vi "Lab Panel V2.3.vi"() -> ()   [LabVIEW 2013]
uses:
  <vilib>/Platform/TimedLoop/XDataNode/timing_clust.ctl
  <vilib>/Platform/TimedLoop/XDataNode/nitl_modes.ctl
  <vilib>/Platform/TimedLoop/XDataNode/wakeup.ctl
  <vilib>/platform/TimedLoop/XDataNode/XDataNode.xnode
  <vilib>/Platform/TimedLoop/XDataNode/XDNodeRunTimeDep.lvlib
panel:
  out "TEMP update":bool
  out "AI update":bool
  in  "stop":bool
  in  "Tab Control 2":T1(tab)
  out "LAB05-2 (SIG)":T2 {"PF" format="%.2f"; "AMPS" format="%.1f"}
  out "LAB05-1 (SIG)":T2 {"PF" format="%.2f"; "AMPS" format="%.1f"}
  out "LAB04-2 (SIG)":T2 {"PF" format="%.2f"; "AMPS" format="%.1f"}
  out "LAB04-1 (SIG)":T2 {"PF" format="%.2f"; "AMPS" format="%.1f"}
  out "LAB03-2 (SIG)":T2 {"PF" format="%.2f"; "AMPS" format="%.1f"}
  out "LAB03-1 (SIG)":T2 {"PF" format="%.2f"; "AMPS" format="%.1f"}
  out "LAB02-2 (SIG)":T2 {"PF" format="%.2f"; "AMPS" format="%.1f"}
  in  "LAB01-1RUN":bool
  in  "LAB05-1 (O/I)":bool
  in  "LAB05-2 (O/I)":bool
  in  "LAB04-1 (O/I)":bool
  in  "LAB04-2 (O/I)":bool
  in  "LAB02-1 (O/I)":bool
  in  "LAB02-2 (O/I)":bool
  in  "LAB01-2 (O/I)":bool
  in  "LAB01-1 (O/I)":bool
  in  "LAB03-1 (O/I)":bool
  in  "LAB05-2 RUN":bool
  in  "LAB05-1 RUN":bool
  in  "LAB04-2 RUN":bool
  in  "LAB04-1 RUN":bool
  in  "LAB03-2 RUN":bool
  in  "LAB03-1 RUN":bool
  in  "LAB02-2 RUN":bool
  in  "LAB02-1 RUN":bool
  in  "LAB01-2 RUN":bool
  in  "LAB05-2 SELECT":T3(radio)
  in  "LAB05-1 SELECT":T3(radio)
  in  "LAB04-2 SELECT":T3(radio)
  in  "LAB04-1 SELECT":T3(radio)
  in  "LAB03-2 SELECT":T3(radio)
  in  "LAB03-1 SELECT":T3(radio)
  in  "LAB02-2 SELECT":T3(radio)
  in  "LAB02-1 SELECT":T3(radio)
  in  "LAB01-2 SELECT":T3(radio)
  in  "LAB01-1 SELECT":T3(radio)
  in  "LAB03-2 (O/I)":bool
  out "LAB01-1 (SIG)":T2 {"PF" format="%.2f"; "AMPS" format="%.1f"}
  out "LAB01-2 (SIG)":T2 {"PF" format="%.2f"; "AMPS" format="%.1f"}
  out "LAB02-1 (SIG)":T2 {"PF" format="%.2f"; "AMPS" format="%.1f"}
  in  "LAB05 (SETTINGS 1)":T4={"1 Name"="", "1 Description"="", "1 (CYCLES)"=1.0, "1 (T-RISE mins)"=1.0, "1 (T-RISE deg C)"=1.0, "2 Name"="", "2 Description"="", "2 (CYCLES)"=1.0, "2 (T-RISE mins)"=1.0, "2 (T-RISE deg C)"=1.0} {"2 (T-RISE deg C)" min=1.0 max=100.0 step=1.0 format="%#.0f"; "2 (T-RISE mins)" min=0.0 max=1000.0 step=10.0 format="%#.0f"; "2 (CYCLES)" min=0.0 max=100000.0 step=10.0; "1 (T-RISE deg C)" min=1.0 max=100.0 step=1.0 format="%#.0f"; "1 (T-RISE mins)" min=0.0 max=1000.0 step=10.0 format="%#.0f"; "1 (CYCLES)" min=0.0 max=100000.0 step=10.0}
  in  "LAB04 (SETTINGS 1)":T4={"1 Name"="", "1 Description"="", "1 (CYCLES)"=1.0, "1 (T-RISE mins)"=1.0, "1 (T-RISE deg C)"=1.0, "2 Name"="", "2 Description"="", "2 (CYCLES)"=1.0, "2 (T-RISE mins)"=1.0, "2 (T-RISE deg C)"=1.0} {"2 (T-RISE deg C)" min=1.0 max=100.0 step=1.0 format="%#.0f"; "2 (T-RISE mins)" min=0.0 max=1000.0 step=10.0 format="%#.0f"; "2 (CYCLES)" min=0.0 max=100000.0 step=10.0; "1 (T-RISE deg C)" min=1.0 max=100.0 step=1.0 format="%#.0f"; "1 (T-RISE mins)" min=0.0 max=1000.0 step=10.0 format="%#.0f"; "1 (CYCLES)" min=0.0 max=100000.0 step=10.0}
  in  "LAB03 (SETTINGS 1)":T4={"1 Name"="", "1 Description"="", "1 (CYCLES)"=1.0, "1 (T-RISE mins)"=1.0, "1 (T-RISE deg C)"=1.0, "2 Name"="", "2 Description"="", "2 (CYCLES)"=1.0, "2 (T-RISE mins)"=1.0, "2 (T-RISE deg C)"=1.0} {"2 (T-RISE deg C)" min=1.0 max=100.0 step=1.0 format="%#.0f"; "2 (T-RISE mins)" min=0.0 max=1000.0 step=10.0 format="%#.0f"; "2 (CYCLES)" min=0.0 max=100000.0 step=10.0; "1 (T-RISE deg C)" min=1.0 max=100.0 step=1.0 format="%#.0f"; "1 (T-RISE mins)" min=0.0 max=1000.0 step=10.0 format="%#.0f"; "1 (CYCLES)" min=0.0 max=100000.0 step=10.0}
  out "LAB05 (DISP 1)":T5 {"2 (T-RISE min)" format="%#.0f"; "2 (CYCLE)" format="%#.0f"; "1 (T-RISE min)" format="%#.0f"; "1 (CYCLE)" format="%#.0f"}
  out "LAB04 (DISP 1)":T5 {"2 (T-RISE min)" format="%#.0f"; "2 (CYCLE)" format="%#.0f"; "1 (T-RISE min)" format="%#.0f"; "1 (CYCLE)" format="%#.0f"}
  out "LAB03 (DISP 1)":T5 {"2 (T-RISE min)" format="%#.0f"; "2 (CYCLE)" format="%#.0f"; "1 (T-RISE min)" format="%#.0f"; "1 (CYCLE)" format="%#.0f"}
  out "LAB02 (DISP 1)":T5 {"2 (T-RISE min)" format="%#.0f"; "2 (CYCLE)" format="%#.0f"; "1 (T-RISE min)" format="%#.0f"; "1 (CYCLE)" format="%#.0f"}
  in  "LAB02 (SETTINGS 1)":T4={"1 Name"="", "1 Description"="", "1 (CYCLES)"=1.0, "1 (T-RISE mins)"=1.0, "1 (T-RISE deg C)"=1.0, "2 Name"="", "2 Description"="", "2 (CYCLES)"=1.0, "2 (T-RISE mins)"=1.0, "2 (T-RISE deg C)"=1.0} {"2 (T-RISE deg C)" min=1.0 max=100.0 step=1.0 format="%#.0f"; "2 (T-RISE mins)" min=0.0 max=1000.0 step=10.0 format="%#.0f"; "2 (CYCLES)" min=0.0 max=100000.0 step=10.0; "1 (T-RISE deg C)" min=1.0 max=100.0 step=1.0 format="%#.0f"; "1 (T-RISE mins)" min=0.0 max=1000.0 step=10.0 format="%#.0f"; "1 (CYCLES)" min=0.0 max=100000.0 step=10.0}
  out "LAB01 (DISP 1)":T5 {"2 (T-RISE min)" format="%#.0f"; "2 (CYCLE)" format="%#.0f"; "1 (T-RISE min)" format="%.2f"; "1 (CYCLE)" format="%#.0f"}
  in  "LAB01 (SETTINGS 1)":T4={"1 Name"="", "1 Description"="", "1 (CYCLES)"=1.0, "1 (T-RISE mins)"=1.0, "1 (T-RISE deg C)"=1.0, "2 Name"="", "2 Description"="", "2 (CYCLES)"=1.0, "2 (T-RISE mins)"=1.0, "2 (T-RISE deg C)"=1.0} {"2 (T-RISE deg C)" min=1.0 max=100.0 step=1.0 format="%#.0f"; "2 (T-RISE mins)" min=0.0 max=1000.0 step=10.0 format="%#.0f"; "2 (CYCLES)" min=0.0 max=100000.0 step=10.0; "1 (T-RISE deg C)" min=1.0 max=100.0 step=1.0 format="%#.0f"; "1 (T-RISE mins)" min=1.0 max=1000.0 step=10.0 format="%#.0f"; "1 (CYCLES)" min=1.0 max=100000.0 step=10.0}
  out "LAB05 (TEMP START)":T6
  out "LAB04 (TEMP START)":T6
  out "LAB03 (TEMP START)":T6
  out "LAB02 (TEMP START)":T6
  out "LAB01 (TEMP START)":T6
  in  "JIG ON TIME (S)":dbl=1.0 min=1.0 max=10.0 step=0.5 format="%.1g"
  in  "JIG OFF TIME (S)":dbl=2.0 min=2.0 max=10.0 step=0.5 format="%.1g"
  out "LAB01-1 (JIG)":bool
  out "LAB01-2 (JIG)":bool
  out "LAB02-1 (JIG)":bool
  out "LAB02-2 (JIG)":bool
  out "LAB03-1 (JIG)":bool
  out "LAB03-2 (JIG)":bool
  out "LAB04-1 (JIG)":bool
  out "LAB04-2 (JIG)":bool
  out "LAB05-1 (JIG)":bool
  out "LAB05-2 (JIG)":bool
  out "LAB01 (CAL)":T7 {"2 (TN) cal" min=0.0 step=0.01 format="%.2f"; "2 (TL) cal" min=0.0 step=0.01 format="%.2f"; "2 (PF) cal" min=0.0 step=0.01 format="%.2f"; "2 (V) cal" min=0.0 step=0.01 format="%.2f"; "2 (A) cal" min=0.0 step=0.01 format="%.2f"; "1 (TN) cal" min=0.0 step=0.01 format="%.2f"; "1 (TL) cal" min=0.0 step=0.01 format="%.2f"; "1 (PF) cal" min=0.0 step=0.01 format="%.2f"; "1 (V) cal" min=0.0 step=0.01 format="%.2f"; "1  (A) cal" min=0.0 step=0.01 format="%.2f"}
  out "LAB03 (CAL)":T7 {"2 (TN) cal" min=0.0 step=0.01 format="%.2f"; "2 (TL) cal" min=0.0 step=0.01 format="%.2f"; "2 (PF) cal" min=0.0 step=0.01 format="%.2f"; "2 (V) cal" min=0.0 step=0.01 format="%.2f"; "2 (A) cal" min=0.0 step=0.01 format="%.2f"; "1 (TN) cal" min=0.0 step=0.01 format="%.2f"; "1 (TL) cal" min=0.0 step=0.01 format="%.2f"; "1 (PF) cal" min=0.0 step=0.01 format="%.2f"; "1 (V) cal" min=0.0 step=0.01 format="%.2f"; "1  (A) cal" min=0.0 step=0.01 format="%.2f"}
  out "LAB02 (CAL)":T8 {"2 (TN) cal" min=0.0 step=0.01 format="%.2f"; "2 (TL) cal" min=0.0 step=0.01 format="%.2f"; "2 (PF) cal" min=0.0 step=0.01 format="%.2f"; "2 (V) cal" min=0.0 step=0.01 format="%.2f"; "2 (A) cal" min=0.0 step=0.01 format="%.2f"; "1 (TN) cal" min=0.0 step=0.01 format="%.2f"; "1 (TL) cal" min=0.0 step=0.01 format="%.2f"; "1 (PF) cal" min=0.0 step=0.01 format="%.2f"; "1 (V) cal" min=0.0 step=0.01 format="%.2f"; "1 (A) cal" min=0.0 step=0.01 format="%.2f"}
  out "LAB05 (CAL)":T7 {"2 (TN) cal" min=0.0 step=0.01 format="%.2f"; "2 (TL) cal" min=0.0 step=0.01 format="%.2f"; "2 (PF) cal" min=0.0 step=0.01 format="%.2f"; "2 (V) cal" min=0.0 step=0.01 format="%.2f"; "2 (A) cal" min=0.0 step=0.01 format="%.2f"; "1 (TN) cal" min=0.0 step=0.01 format="%.2f"; "1 (TL) cal" min=0.0 step=0.01 format="%.2f"; "1 (PF) cal" min=0.0 step=0.01 format="%.2f"; "1 (V) cal" min=0.0 step=0.01 format="%.2f"; "1  (A) cal" min=0.0 step=0.01 format="%.2f"}
  out "LAB04 (CAL)":T7 {"2 (TN) cal" min=0.0 step=0.01 format="%.2f"; "2 (TL) cal" min=0.0 step=0.01 format="%.2f"; "2 (PF) cal" min=0.0 step=0.01 format="%.2f"; "2 (V) cal" min=0.0 step=0.01 format="%.2f"; "2 (A) cal" min=0.0 step=0.01 format="%.2f"; "1 (TN) cal" min=0.0 step=0.01 format="%.2f"; "1 (TL) cal" min=0.0 step=0.01 format="%.2f"; "1 (PF) cal" min=0.0 step=0.01 format="%.2f"; "1 (V) cal" min=0.0 step=0.01 format="%.2f"; "1  (A) cal" min=0.0 step=0.01 format="%.2f"}
  out "calibration file error out":errorcluster
  in  "CALIBRATE":bool
  in  "Tab Control":T9(tab)
  out "LAB01-2 (GRAPH)":dynamicdata(graph)
  out "LAB01-1 (GRAPH)":dynamicdata(graph)
  out "LAB02-2 (GRAPH)":dynamicdata(graph)
  out "LAB02-1 (GRAPH)":dynamicdata(graph)
  out "LAB03-2 (GRAPH)":dynamicdata(graph)
  out "LAB03-1 (GRAPH)":dynamicdata(graph)
  out "LAB04-2 (GRAPH)":dynamicdata(graph)
  out "LAB04-1 (GRAPH)":dynamicdata(graph)
  out "LAB05-2 (GRAPH)":dynamicdata(graph)
  out "LAB05-1 (GRAPH)":dynamicdata(graph)
  out "LAB05 TEMP":T10
  out "LAB04 TEMP":T10
  out "LAB02 TEMP":T10
  out "LAB01 TEMP":T10
  out "LAB03 TEMP":T10
  out "Analog Error Array":errorcluster[](array[cluster])
  out "AI loop time":dbl format="%.6g"
  out "loops":dbl
  in  "loop  delay(mS)":dbl
  out "on loops":dbl
  out "off loops":dbl
  out "jig cycle":dbl
  out "LAB01-1 (TDMS)":refnum<k34>
  out "LAB01-2 (TDMS)":refnum<k34>
  out "data file error":errorcluster
  # "LAB01"
  # "LAB02"
  # "LAB05"
  # "LAB03"
  # "LAB04"
  # "LAB01"
  # "LAB02"
  # "LAB03"
  # "LAB04"
  # "LAB05"
  # "JIG SET"
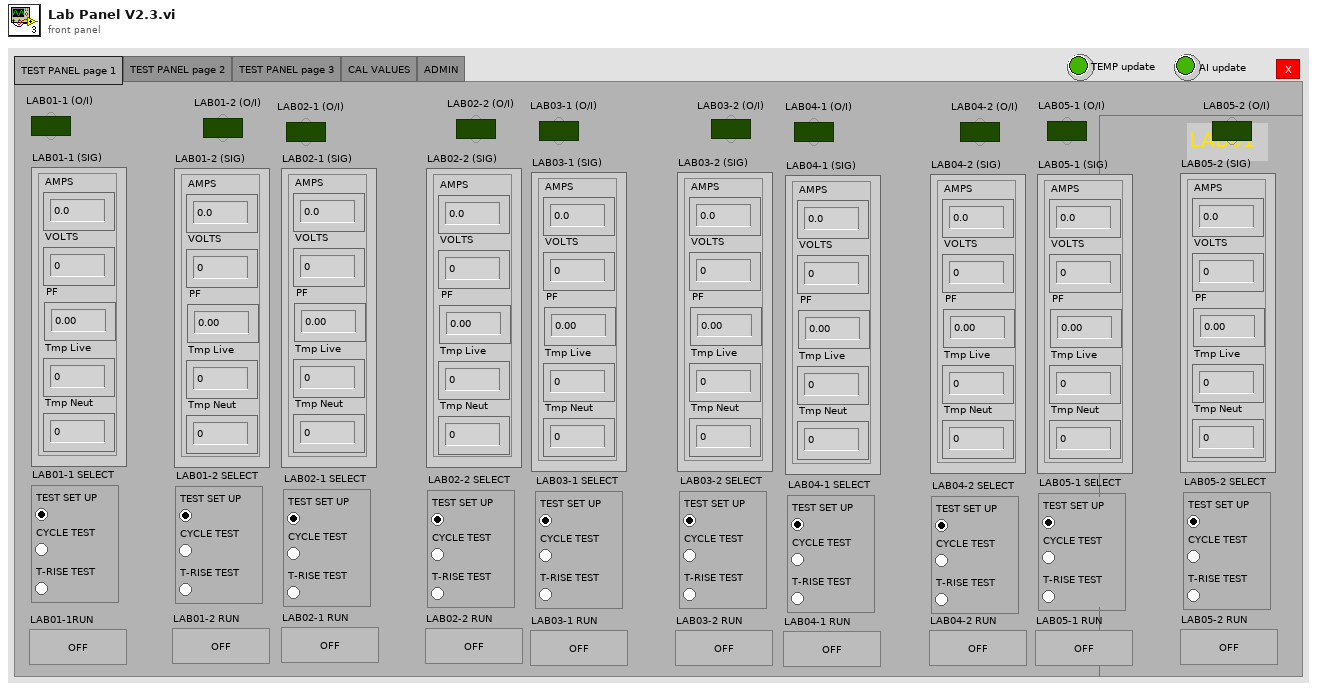
[diagram p1: front panel]
types:
  T1 = enum32{"TEST PANEL page 1", "TEST PANEL page 2", "TEST PANEL page 3", "CAL VALUES", "ADMIN"}
  T2 = cluster{"AMPS":dbl, "VOLTS":dbl, "PF":dbl, "Tmp Live":dbl, "Tmp Neut":dbl}
  T3 = enum32{"TEST SET UP", "CYCLE TEST", "T-RISE TEST"}
  T4 = cluster{"1 Name":string, "1 Description":string, "1 (CYCLES)":dbl, "1 (T-RISE mins)":dbl, "1 (T-RISE deg C)":dbl, "2 Name":string, "2 Description":string, "2 (CYCLES)":dbl, "2 (T-RISE mins)":dbl, "2 (T-RISE deg C)":dbl}
  T5 = cluster{"1 (CYCLE)":dbl, "1 (T-RISE min)":dbl, "1 (STATUS)":string, "2 (CYCLE)":dbl, "2 (T-RISE min)":dbl, "2 (STATUS)":string}
  T6 = cluster{"1 (TL)":dbl, "1 (TN)":dbl, "2 (TL)":dbl, "2 (TN)":dbl}
  T7 = cluster{"1  (A) cal":dbl, "1 (V) cal":dbl, "1 (PF) cal":dbl, "1 (TL) cal":dbl, "1 (TN) cal":dbl, "2 (A) cal":dbl, "2 (V) cal":dbl, "2 (PF) cal":dbl, "2 (TL) cal":dbl, "2 (TN) cal":dbl}
  T8 = cluster{"1 (A) cal":dbl, "1 (V) cal":dbl, "1 (PF) cal":dbl, "1 (TL) cal":dbl, "1 (TN) cal":dbl, "2 (A) cal":dbl, "2 (V) cal":dbl, "2 (PF) cal":dbl, "2 (TL) cal":dbl, "2 (TN) cal":dbl}
  T9 = enum32{"LAB01", "LAB02", "LAB03", "LAB04", "LAB05", "TEMPERATURE", "ERROR"}
  T10 = cluster{"T1 Live":dbl, "T1 Neut":dbl, "T2 Live":dbl, "T2 Neut":dbl, "ID":dbl, "ER":dbl}
  T11 = typedef "XDNodeRunTimeDep.lvlib/timing_clust.ctl" = cluster{"Expected End [f-1]":u64, "Actual End [f-1]":u64, "Finished Late? [f-1]":bool, "Expected End [i-1]":u64, "Actual End [i-1]":u64, "Finished Late? [i-1]":bool, "Expected Start [i]":u64, "Actual Start [i]":u64, "Expected Start [f]":u64, "Actual Start [f]":u64, "Source Name":string, "Structure Name":string, "Period":i64, "Deadline":i64, "Offset":i64, "Start":i64, "Priority":i32, "Timeout":i32, "Mode":T12, "Wakeup Reason":T13, "Error":errorcluster, "Source Type":string, "Secondary Source Type":string, "Global End Time":u64, "Global Start Time":u64, "Frame Duration":u64, "Iteration Duration":u64, "Assigned CPU":i32, "I/O Scan Engine Mode":u32}
  T12 = typedef "XDNodeRunTimeDep.lvlib/nitl_modes.ctl" = enum32{"No Change", "Process missed periods, maintain original phase", "Discard missed periods, maintain original phase", "Process missed periods, ignore original phase", "Discard missed periods, ignore original phase"}
  T13 = typedef "XDNodeRunTimeDep.lvlib/wakeup.ctl" = enum32{"Normal", "Aborted", "Asynchronous wakeup", "Timing source error", "Timed loop error", "Timeout"}
  T14 = enum16{"open", "open or create", "create or replace", "create", "open (read-only)"}
  T15 = cluster{"T1":dbl, "T2":dbl, "T3":dbl, "T4":dbl, "ID":dbl, "ER":dbl}
  T16 = cluster{"LAB01-1 (A)":dbl, "LAB01-1 (V)":dbl, "LAB01-1 (PF)":dbl, "LAB01-2 (A)":dbl, "LAB01-2 (V)":dbl, "LAB01-2 (PF)":dbl}
  T17 = cluster{"LAB02-1 (A)":dbl, "LAB02-1 (V)":dbl, "LAB02-1 (PF)":dbl, "LAB02-2 (A)":dbl, "LAB02-2 (V)":dbl, "LAB02-2 (PF)":dbl}
  T18 = cluster{"LAB03-1 (A)":dbl, "LAB03-1 (V)":dbl, "LAB03-1 (PF)":dbl, "LAB03-2 (A)":dbl, "LAB03-2 (V)":dbl, "LAB03-2 (PF)":dbl}
  T19 = cluster{"LAB04-1 (A)":dbl, "LAB04-1 (V)":dbl, "LAB04-1 (PF)":dbl, "LAB04-2 (A)":dbl, "LAB04-2 (V)":dbl, "LAB04-2 (PF)":dbl}
  T20 = cluster{"LAB05-1 (A)":dbl, "LAB05-1 (V)":dbl, "LAB05-1 (PF)":dbl, "LAB05-2 (A)":dbl, "LAB05-2 (V)":dbl, "LAB05-2 (PF)":dbl}
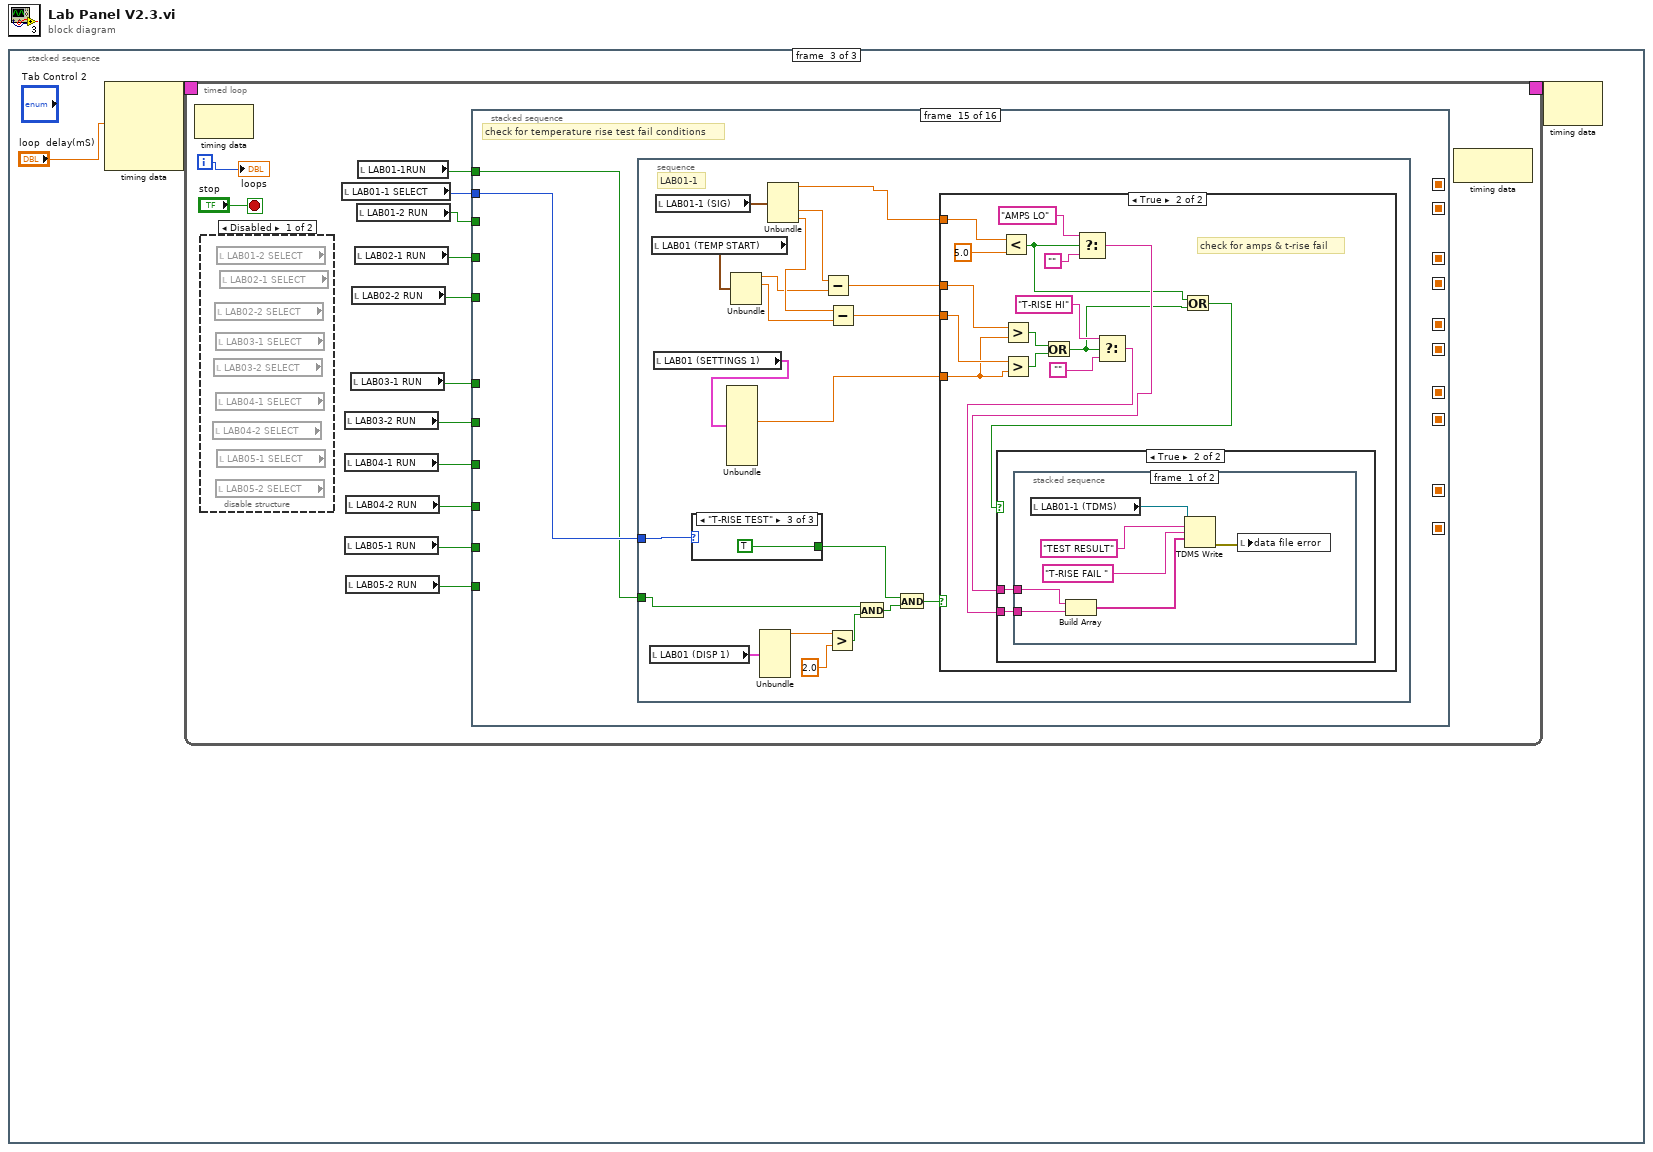
[diagram p0: block diagram]
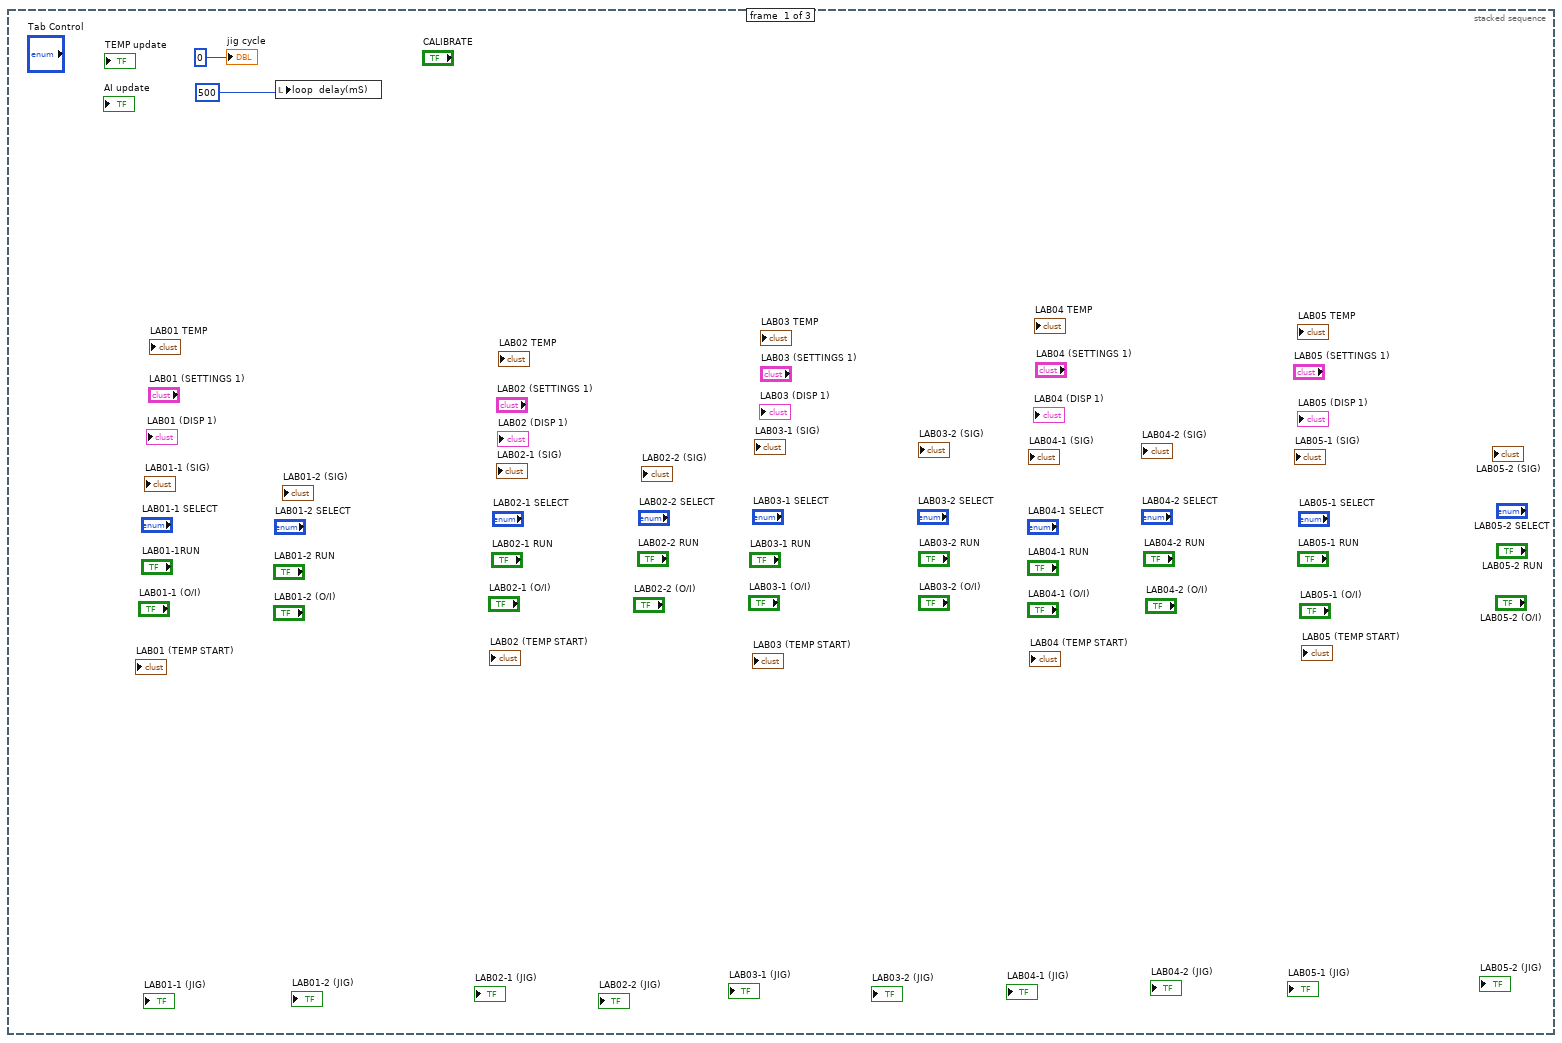
[diagram p2: hidden frame]
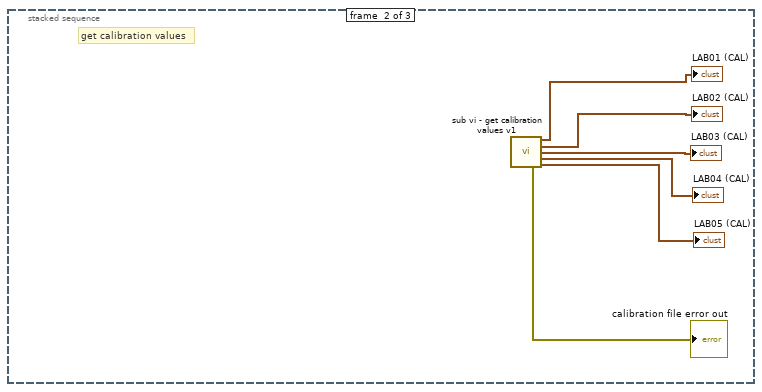
[diagram p3: hidden frame]
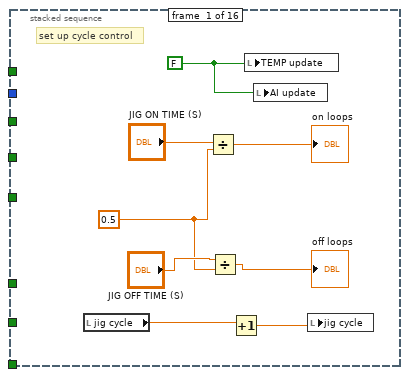
[diagram p5: hidden frame]
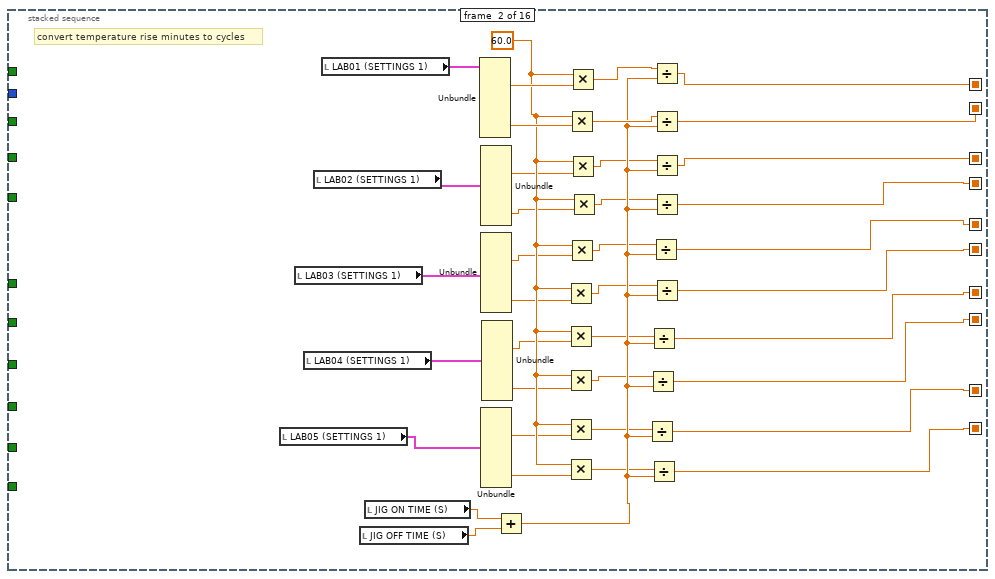
[diagram p6: hidden frame]
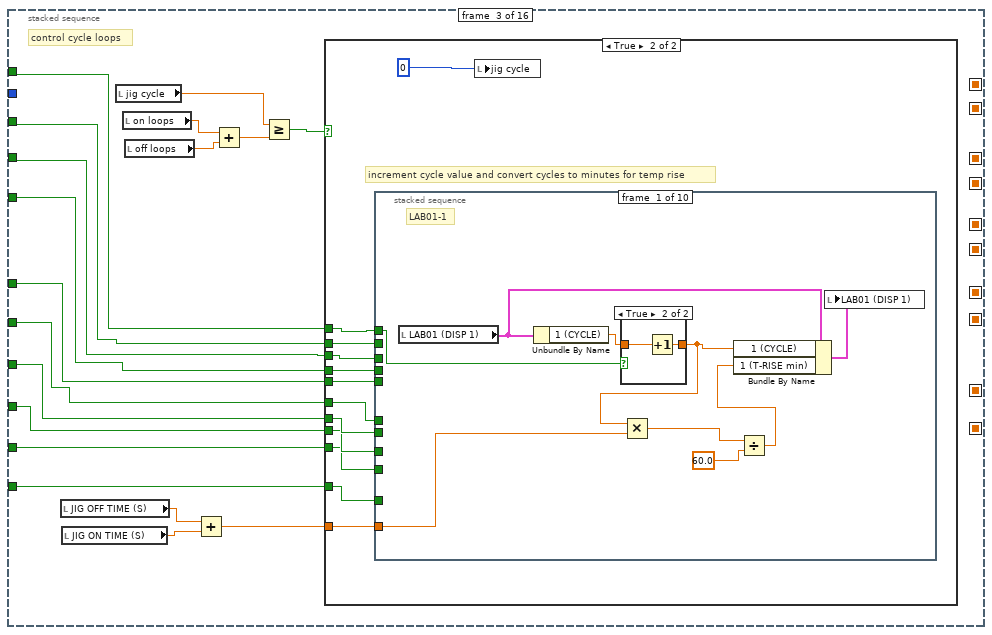
[diagram p7: hidden frame]
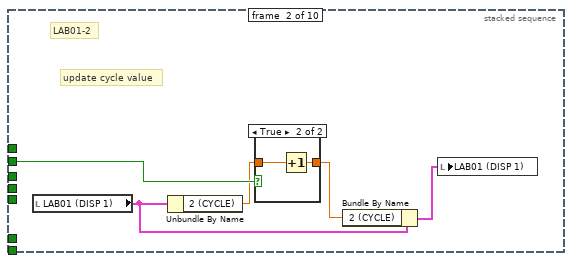
[diagram p10: hidden frame]
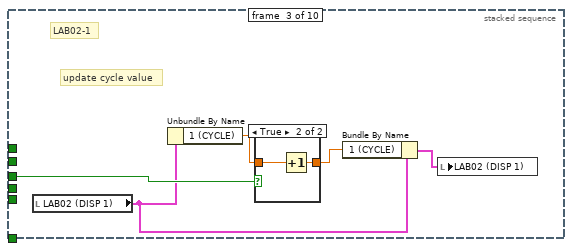
[diagram p12: hidden frame]
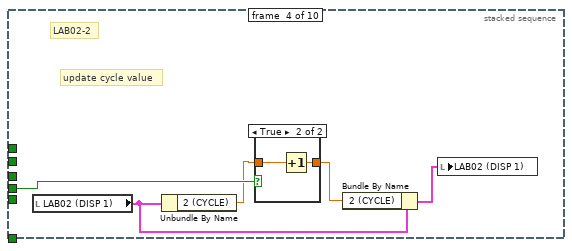
[diagram p14: hidden frame]
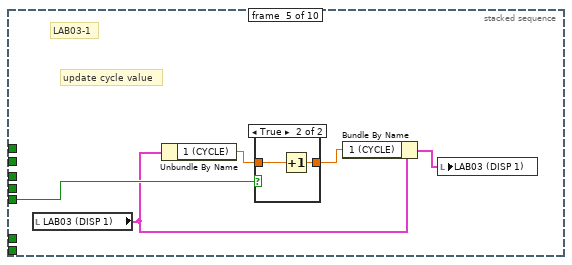
[diagram p16: hidden frame]
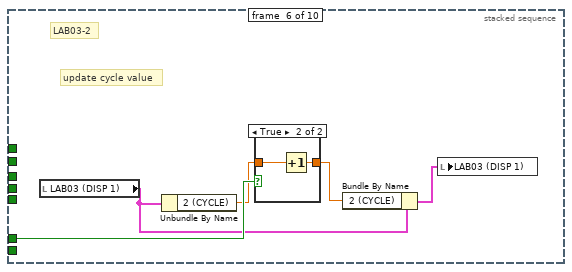
[diagram p18: hidden frame]
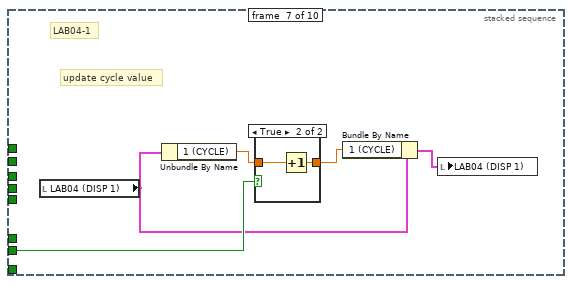
[diagram p20: hidden frame]
diagram:
  n1 = stacked-sequence {
    frame #0 {
      n2 = local write "loop  delay(mS)"(500) -> ()
      "jig cycle" <- 0
    }
    frame #1 {
      # "get calibration values"
      n3 = call "sub vi - get calibration values v1.vi"() -> ("LAB01 (CAL)"=→"LAB01 (CAL)":T7, "LAB02 (CAL)"=→"LAB02 (CAL)":T8, "LAB03 (CAL)"=→"LAB03 (CAL)":T7, "LAB04 (CAL)"=→"LAB04 (CAL)":T7, "calibration file error out"=→"calibration file error out":errorcluster, "LAB05 (CAL)"=→"LAB05 (CAL)":T7)  [unwired: 10 in]
    }
    frame #2 {
      n4 = node-c288("loop  delay(mS)") -> (w11:T11)  [unwired: 3 in]
      n5 = timed-loop {
        timing: w11 -> [_]
        timing-out: [_] -> w10
        i -> [w24]
        stop <- "stop" stop-if-true
        n6 = node-c288() -> ()  [unwired: 1 in, 1 out]
        n7 = disable-structure shown="Disabled" {
          frame Disabled {
            n8 = local read "LAB04-2 SELECT"() -> ()  [unwired: 1 out]
            n9 = local read "LAB03-2 SELECT"() -> ()  [unwired: 1 out]
            n10 = local read "LAB02-2 SELECT"() -> ()  [unwired: 1 out]
            n11 = local read "LAB03-1 SELECT"() -> ()  [unwired: 1 out]
            n12 = local read "LAB04-1 SELECT"() -> ()  [unwired: 1 out]
            n13 = local read "LAB05-2 SELECT"() -> ()  [unwired: 1 out]
            n14 = local read "LAB01-2 SELECT"() -> ()  [unwired: 1 out]
            n15 = local read "LAB05-1 SELECT"() -> ()  [unwired: 1 out]
            n16 = local read "LAB02-1 SELECT"() -> ()  [unwired: 1 out]
          }
          frame Enabled {
          }
        }
        n17 = local read "LAB01-1 SELECT"() -> (w12:T3)
        n18 = local read "LAB03-2 RUN"() -> (w17:bool)
        n19 = local read "LAB04-1 RUN"() -> (w16:bool)
        n20 = local read "LAB05-1 RUN"() -> (w14:bool)
        n21 = local read "LAB04-2 RUN"() -> (w15:bool)
        n22 = local read "LAB05-2 RUN"() -> (w13:bool)
        n23 = local read "LAB03-1 RUN"() -> (w18:bool)
        n24 = local read "LAB02-2 RUN"() -> (w19:bool)
        n25 = local read "LAB02-1 RUN"() -> (w20:bool)
        n26 = local read "LAB01-2 RUN"() -> (w21:bool)
        n27 = local read "LAB01-1RUN"() -> (w22:bool)
        n28 = stacked-sequence {
          seq-local: [_ w70 _ _ _ _ _ _ _ _ _ _ _ _ _ _] -> [_ _ _ _ w234 _ _ _ _ _ _ _ _ _ _ _]
          seq-local: [_ w69 _ _ _ _ _ _ _ _ _ _ _ _ _ _] -> [_ _ _ _ _ _ _ _ _ _ _ _ _ _ _ _]
          seq-local: [_ w42 _ _ _ _ _ _ _ _ _ _ _ _ _ _] -> [_ _ _ _ _ _ _ _ _ _ _ _ _ _ _ _]
          seq-local: [_ w41 _ _ _ _ _ _ _ _ _ _ _ _ _ _] -> [_ _ _ _ _ _ _ _ _ _ _ _ _ _ _ _]
          seq-local: [_ w40 _ _ _ _ _ _ _ _ _ _ _ _ _ _] -> [_ _ _ _ _ _ _ _ _ _ _ _ _ _ _ _]
          seq-local: [_ w39 _ _ _ _ _ _ _ _ _ _ _ _ _ _] -> [_ _ _ _ _ _ _ _ _ _ _ _ _ _ _ _]
          seq-local: [_ w38 _ _ _ _ _ _ _ _ _ _ _ _ _ _] -> [_ _ _ _ _ _ _ _ _ _ _ _ _ _ _ _]
          seq-local: [_ w37 _ _ _ _ _ _ _ _ _ _ _ _ _ _] -> [_ _ _ _ _ _ _ _ _ _ _ _ _ _ _ _]
          seq-local: [_ w36 _ _ _ _ _ _ _ _ _ _ _ _ _ _] -> [_ _ _ _ _ _ _ _ _ _ _ _ _ _ _ _]
          seq-local: [_ w35 _ _ _ _ _ _ _ _ _ _ _ _ _ _] -> [_ _ _ _ _ _ _ _ _ _ _ _ _ _ _ _]
          tunnel: w22 -> [_ _ w87 w198 w245 w281 w344 _ _ _ _ _ w806 w862 w920 _]
          tunnel: w21 -> [_ _ w86 w197 w244 w280 _ _ _ _ _ _ _ _ _ _]
          tunnel: w20 -> [_ _ w85 w196 w243 w279 _ _ _ _ _ _ _ _ _ _]
          tunnel: w19 -> [_ _ w84 w195 w242 w278 _ _ _ _ _ _ _ _ _ _]
          tunnel: w18 -> [_ _ w83 w194 w241 w277 _ _ _ _ _ _ _ _ _ _]
          tunnel: w17 -> [_ _ w82 w193 w240 w276 _ _ _ _ _ _ _ _ _ _]
          tunnel: w16 -> [_ _ w81 w192 w239 w275 _ _ _ _ _ _ _ _ _ _]
          tunnel: w15 -> [_ _ w80 w191 w238 w274 _ _ _ _ _ _ _ _ _ _]
          tunnel: w14 -> [_ _ w79 w190 w237 w273 _ _ _ _ _ _ _ _ _ _]
          tunnel: w13 -> [_ _ w78 w189 w236 w272 _ _ _ _ _ _ _ _ _ _]
          tunnel: w12 -> [_ _ _ w188 w235 _ w345 _ _ _ _ _ _ w864 w921 _]
          frame #0 {
            w27 = FALSE
            w32 = 0.5
            # "set up cycle control"
            n29 = local read "jig cycle"() -> (w31:dbl)
            n30 = Divide(x="JIG ON TIME (S)", y=w32) -> (x/y=→"on loops":dbl)
            n31 = Divide(x="JIG OFF TIME (S)", y=w32) -> (x/y=→"off loops":dbl)
            n32 = Increment(x=w31) -> (x+1=w30:dbl)
            n33 = local write "TEMP update"(w27) -> ()
            n34 = local write "AI update"(w27) -> ()
            n35 = local write "jig cycle"(w30) -> ()
          }
          frame #1 {
            w60 = 60.0
            # "convert temperature rise minutes to cycles"
            n36 = local read "LAB05 (SETTINGS 1)"() -> (w61:T4)
            n37 = local read "LAB03 (SETTINGS 1)"() -> (w63:T4)
            n38 = local read "LAB04 (SETTINGS 1)"() -> (w62:T4)
            n39 = local read "LAB02 (SETTINGS 1)"() -> (w64:T4)
            n40 = local read "LAB01 (SETTINGS 1)"() -> (w73:T4)
            n41 = local read "JIG OFF TIME (S)"() -> (w71:dbl)
            n42 = local read "JIG ON TIME (S)"() -> (w72:dbl)
            n43 = Unbundle(w73) -> ("1 (T-RISE mins)"=w68:dbl, "2 (T-RISE mins)"=w67:dbl)  [unwired: 8 out]
            n44 = Unbundle(w64) -> ("1 (T-RISE mins)"=w59:dbl, "2 (T-RISE mins)"=w58:dbl)  [unwired: 8 out]
            n45 = Unbundle(w63) -> ("1 (T-RISE mins)"=w57:dbl, "2 (T-RISE mins)"=w56:dbl)  [unwired: 8 out]
            n46 = Unbundle(w61) -> ("1 (T-RISE mins)"=w53:dbl, "2 (T-RISE mins)"=w52:dbl)  [unwired: 8 out]
            n47 = Unbundle(w62) -> ("1 (T-RISE mins)"=w55:dbl, "2 (T-RISE mins)"=w54:dbl)  [unwired: 8 out]
            n48 = Add(x=w72, y=w71) -> (x+y=w51:dbl)
            n49 = Multiply(x=w60, y=w56) -> (x*y=w47:dbl)
            n50 = Multiply(x=w60, y=w55) -> (x*y=w46:dbl)
            n51 = Multiply(x=w60, y=w54) -> (x*y=w45:dbl)
            n52 = Multiply(x=w60, y=w53) -> (x*y=w44:dbl)
            n53 = Multiply(x=w60, y=w52) -> (x*y=w43:dbl)
            n54 = Multiply(x=w60, y=w67) -> (x*y=w65:dbl)
            n55 = Multiply(x=w60, y=w57) -> (x*y=w48:dbl)
            n56 = Multiply(x=w60, y=w68) -> (x*y=w66:dbl)
            n57 = Multiply(x=w60, y=w59) -> (x*y=w50:dbl)
            n58 = Multiply(x=w60, y=w58) -> (x*y=w49:dbl)
            n59 = Divide(x=w44, y=w51) -> (x/y=w36:dbl)
            n60 = Divide(x=w45, y=w51) -> (x/y=w37:dbl)
            n61 = Divide(x=w46, y=w51) -> (x/y=w38:dbl)
            n62 = Divide(x=w43, y=w51) -> (x/y=w35:dbl)
            n63 = Divide(x=w48, y=w51) -> (x/y=w40:dbl)
            n64 = Divide(x=w66, y=w51) -> (x/y=w70:dbl)
            n65 = Divide(x=w65, y=w51) -> (x/y=w69:dbl)
            n66 = Divide(x=w50, y=w51) -> (x/y=w42:dbl)
            n67 = Divide(x=w49, y=w51) -> (x/y=w41:dbl)
            n68 = Divide(x=w47, y=w51) -> (x/y=w39:dbl)
          }
          frame #2 {
            # "control cycle loops"
            n69 = local read "JIG OFF TIME (S)"() -> (w76:dbl)
            n70 = local read "JIG ON TIME (S)"() -> (w75:dbl)
            n71 = local read "jig cycle"() -> (w89:dbl)
            n72 = local read "on loops"() -> (w91:dbl)
            n73 = local read "off loops"() -> (w90:dbl)
            n74 = Add(x=w76, y=w75) -> (x+y=w74:dbl)
            n75 = Add(x=w91, y=w90) -> (x+y=w77:dbl)
            n76 = Greater Or Equal?(x=w89, y=w77) -> (x >= y?=w88:bool)
            n77 = case shown="True" w88 {
              tunnel: w87 -> [_ w102]
              tunnel: w86 -> [_ w101]
              tunnel: w85 -> [_ w100]
              tunnel: w84 -> [_ w99]
              tunnel: w83 -> [_ w98]
              tunnel: w82 -> [_ w97]
              tunnel: w81 -> [_ w96]
              tunnel: w80 -> [_ w95]
              tunnel: w79 -> [_ w94]
              tunnel: w78 -> [_ w93]
              tunnel: w74 -> [_ w92]
              frame False {
              }
              frame True {
                # "increment cycle value and convert cycles to minutes for temp rise"
                n78 = stacked-sequence {
                  tunnel: w102 -> [w112 _ _ _ _ _ _ _ _ _]
                  tunnel: w101 -> [_ w120 _ _ _ _ _ _ _ _]
                  tunnel: w100 -> [_ _ w128 _ _ _ _ _ _ _]
                  tunnel: w99 -> [_ _ _ w136 _ _ _ _ _ _]
                  tunnel: w98 -> [_ _ _ _ w144 _ _ _ _ _]
                  tunnel: w97 -> [_ _ _ _ _ w152 _ _ _ _]
                  tunnel: w96 -> [_ _ _ _ _ _ w160 _ _ _]
                  tunnel: w95 -> [_ _ _ _ _ _ _ w168 _ _]
                  tunnel: w94 -> [_ _ _ _ _ _ _ _ w176 _]
                  tunnel: w93 -> [_ _ _ _ _ _ _ _ _ w184]
                  tunnel: w92 -> [w104 _ _ _ _ _ _ _ _ _]
                  frame #0 {
                    # "LAB01-1"
                    n79 = local read "LAB01 (DISP 1)"() -> (w109:T5)
                    n80 = Unbundle By Name(w109) -> ("1 (CYCLE)"=w110:dbl)
                    n81 = case shown="True" w112 {
                      tunnel: w110 -> [w113 w115]
                      tunnel: [w113 w114] -> w106
                      frame False {
                      }
                      frame True {
                        n82 = Increment(x=w115) -> (x+1=w114:dbl)
                      }
                    }
                    n83 = Multiply(x=w106, y=w104) -> (x*y=w105:dbl)
                    n84 = Divide(x=w105, y=60.0) -> (x/y=w107:dbl)
                    n85 = Bundle By Name(cluster=w109, "1 (CYCLE)"=w106, "1 (T-RISE min)"=w107) -> (w111:T5)
                    n86 = local write "LAB01 (DISP 1)"(w111) -> ()
                  }
                  frame #1 {
                    # "update cycle value"
                    # "LAB01-2"
                    n87 = local read "LAB01 (DISP 1)"() -> (w118:T5)
                    n88 = Unbundle By Name(w118) -> ("2 (CYCLE)"=w117:dbl)
                    n89 = case shown="True" w120 {
                      tunnel: w117 -> [w121 w123]
                      tunnel: [w121 w122] -> w116
                      frame False {
                      }
                      frame True {
                        n90 = Increment(x=w123) -> (x+1=w122:dbl)
                      }
                    }
                    n91 = Bundle By Name(cluster=w118, "2 (CYCLE)"=w116) -> (w119:T5)
                    n92 = local write "LAB01 (DISP 1)"(w119) -> ()
                  }
                  frame #2 {
                    # "update cycle value"
                    # "LAB02-1"
                    n93 = local read "LAB02 (DISP 1)"() -> (w126:T5)
                    n94 = Unbundle By Name(w126) -> ("1 (CYCLE)"=w124:dbl)
                    n95 = case shown="True" w128 {
                      tunnel: [w129 w131] -> w125
                      tunnel: w124 -> [w129 w130]
                      frame False {
                      }
                      frame True {
                        n96 = Increment(x=w130) -> (x+1=w131:dbl)
                      }
                    }
                    n97 = Bundle By Name(cluster=w126, "1 (CYCLE)"=w125) -> (w127:T5)
                    n98 = local write "LAB02 (DISP 1)"(w127) -> ()
                  }
                  frame #3 {
                    # "update cycle value"
                    # "LAB02-2"
                    n99 = local read "LAB02 (DISP 1)"() -> (w134:T5)
                    n100 = Unbundle By Name(w134) -> ("2 (CYCLE)"=w133:dbl)
                    n101 = case shown="True" w136 {
                      tunnel: [w137 w139] -> w132
                      tunnel: w133 -> [w137 w138]
                      frame False {
                      }
                      frame True {
                        n102 = Increment(x=w138) -> (x+1=w139:dbl)
                      }
                    }
                    n103 = Bundle By Name(cluster=w134, "2 (CYCLE)"=w132) -> (w135:T5)
                    n104 = local write "LAB02 (DISP 1)"(w135) -> ()
                  }
                  frame #4 {
                    # "update cycle value"
                    # "LAB03-1"
                    n105 = local read "LAB03 (DISP 1)"() -> (w142:T5)
                    n106 = Unbundle By Name(w142) -> ("1 (CYCLE)"=w141:dbl)
                    n107 = case shown="True" w144 {
                      tunnel: [w145 w147] -> w140
                      tunnel: w141 -> [w145 w146]
                      frame False {
                      }
                      frame True {
                        n108 = Increment(x=w146) -> (x+1=w147:dbl)
                      }
                    }
                    n109 = Bundle By Name(cluster=w142, "1 (CYCLE)"=w140) -> (w143:T5)
                    n110 = local write "LAB03 (DISP 1)"(w143) -> ()
                  }
                  frame #5 {
                    # "update cycle value"
                    # "LAB03-2"
                    n111 = local read "LAB03 (DISP 1)"() -> (w150:T5)
                    n112 = Unbundle By Name(w150) -> ("2 (CYCLE)"=w149:dbl)
                    n113 = case shown="True" w152 {
                      tunnel: [w153 w155] -> w148
                      tunnel: w149 -> [w153 w154]
                      frame False {
                      }
                      frame True {
                        n114 = Increment(x=w154) -> (x+1=w155:dbl)
                      }
                    }
                    n115 = Bundle By Name(cluster=w150, "2 (CYCLE)"=w148) -> (w151:T5)
                    n116 = local write "LAB03 (DISP 1)"(w151) -> ()
                  }
                  frame #6 {
                    # "update cycle value"
                    # "LAB04-1"
                    n117 = local read "LAB04 (DISP 1)"() -> (w158:T5)
                    n118 = Unbundle By Name(w158) -> ("1 (CYCLE)"=w157:dbl)
                    n119 = case shown="True" w160 {
                      tunnel: [w161 w163] -> w156
                      tunnel: w157 -> [w161 w162]
                      frame False {
                      }
                      frame True {
                        n120 = Increment(x=w162) -> (x+1=w163:dbl)
                      }
                    }
                    n121 = Bundle By Name(cluster=w158, "1 (CYCLE)"=w156) -> (w159:T5)
                    n122 = local write "LAB04 (DISP 1)"(w159) -> ()
                  }
                  frame #7 {
                    # "update cycle value"
                    # "LAB04-2"
                    n123 = local read "LAB04 (DISP 1)"() -> (w166:T5)
                    n124 = Unbundle By Name(w166) -> ("2 (CYCLE)"=w165:dbl)
                    n125 = case shown="True" w168 {
                      tunnel: [w169 w171] -> w164
                      tunnel: w165 -> [w169 w170]
                      frame False {
                      }
                      frame True {
                        n126 = Increment(x=w170) -> (x+1=w171:dbl)
                      }
                    }
                    n127 = Bundle By Name(cluster=w166, "2 (CYCLE)"=w164) -> (w167:T5)
                    n128 = local write "LAB04 (DISP 1)"(w167) -> ()
                  }
                  frame #8 {
                    # "update cycle value"
                    # "LAB05-1"
                    n129 = local read "LAB05 (DISP 1)"() -> (w174:T5)
                    n130 = Unbundle By Name(w174) -> ("1 (CYCLE)"=w173:dbl)
                    n131 = case shown="True" w176 {
                      tunnel: [w177 w179] -> w172
                      tunnel: w173 -> [w177 w178]
                      frame False {
                      }
                      frame True {
                        n132 = Increment(x=w178) -> (x+1=w179:dbl)
                      }
                    }
                    n133 = Bundle By Name(cluster=w174, "1 (CYCLE)"=w172) -> (w175:T5)
                    n134 = local write "LAB05 (DISP 1)"(w175) -> ()
                  }
                  frame #9 {
                    # "update cycle value"
                    # "LAB05-2"
                    n135 = local read "LAB05 (DISP 1)"() -> (w182:T5)
                    n136 = Unbundle By Name(w182) -> ("2 (CYCLE)"=w181:dbl)
                    n137 = case shown="True" w184 {
                      tunnel: [w185 w187] -> w180
                      tunnel: w181 -> [w185 w186]
                      frame False {
                      }
                      frame True {
                        n138 = Increment(x=w186) -> (x+1=w187:dbl)
                      }
                    }
                    n139 = Bundle By Name(cluster=w182, "2 (CYCLE)"=w180) -> (w183:T5)
                    n140 = local write "LAB05 (DISP 1)"(w183) -> ()
                  }
                }
                n141 = local write "jig cycle"(0) -> ()
              }
            }
          }
          frame #3 {
            # "check if test cycles reached for cycle tests, if so then test pass"
            n142 = stacked-sequence {
              tunnel: w198 -> [_]
              tunnel: w197 -> [_]
              tunnel: w196 -> [_]
              tunnel: w195 -> [_]
              tunnel: w194 -> [_]
              tunnel: w193 -> [_]
              tunnel: w192 -> [_]
              tunnel: w191 -> [_]
              tunnel: w190 -> [_]
              tunnel: w189 -> [_]
              tunnel: w188 -> [w203]
              frame #0 {
                # "LAB01-1"
                n143 = Less?(x=w203, y=2) -> (x < y?=w201:bool)
                n144 = local read "LAB01 (DISP 1)"() -> (w204:T5)
                n145 = Unbundle(w204) -> ("1 (STATUS)"=w205:string)  [unwired: 5 out]
                n146 = Equal?(x=w205, y="RUN") -> (x = y?=w200:bool)
                n147 = And(x=w200, y=w201) -> (x .and. y?=w199:bool)
                n148 = case shown="True" w199 {
                  tunnel: w204 -> [_ w212]
                  tunnel: w203 -> [_ w211]
                  frame False {
                  }
                  frame True {
                    n149 = local read "LAB01 (SETTINGS 1)"() -> (w214:T4)
                    n150 = Unbundle(w212) -> ("1 (CYCLE)"=w213:dbl)  [unwired: 5 out]
                    n151 = Unbundle(w214) -> ("1 (CYCLES)"=w208:dbl, "1 (T-RISE mins)"=w210:dbl)  [unwired: 8 out]
                    n152 = case shown="\"TEST SET UP\", Default" w211 {
                      tunnel: w210 -> [_ _ w221]
                      tunnel: [w216 w218 w221] -> w209
                      tunnel: w208 -> [w216 w218 _]
                      tunnel: ["TEST SET UP CYCLES" "CYCLES" "T-RISE TEST"] -> w207
                      frame "TEST SET UP", Default {
                      }
                      frame "CYCLE TEST" {
                      }
                      frame "T-RISE TEST" {
                      }
                    }
                    n153 = Greater Or Equal?(x=w213, y=w208) -> (x >= y?=w215:bool)
                    n154 = case shown="True" w215 {
                      tunnel: w209 -> [w223 _]
                      tunnel: w207 -> [w222 _]
                      frame True {
                        n155 = stacked-sequence {
                          tunnel: w223 -> [w226 _]
                          tunnel: w222 -> [w224 _]
                          frame #0 {
                            n156 = local read "LAB01-1 (TDMS)"() -> (w230:refnum<k34>)
                            n157 = Build Array(w224) -> (w227:string[])
                            n158 = Build Array(w226) -> (w225:dbl[])
                            n159 = TDMS Write(0:w230, 5:"TEST PASS", 7:w227, 9:w225) -> (15:w229:errorcluster)  [unwired: 2 in, 3 out]
                            n160 = local write "data file error"(w229) -> ()
                          }
                          frame #1 {
                            n161 = local read "LAB01 (DISP 1)"() -> (w233:T5)
                            n162 = Bundle(cluster=w233, "1 (STATUS)"="STOP") -> (w231:T5)  [unwired: 5 in]
                            n163 = local write "LAB01 (DISP 1)"(w231) -> ()
                          }
                        }
                      }
                      frame False {
                      }
                    }
                  }
                }
              }
            }
          }
          frame #4 {
            # "check if test cycles reached for temperature rise test"
            n164 = stacked-sequence {
              tunnel: w245 -> [_]
              tunnel: w244 -> [_]
              tunnel: w243 -> [_]
              tunnel: w242 -> [_]
              tunnel: w241 -> [_]
              tunnel: w240 -> [_]
              tunnel: w239 -> [_]
              tunnel: w238 -> [_]
              tunnel: w237 -> [_]
              tunnel: w236 -> [_]
              tunnel: w235 -> [w251]
              tunnel: w234 -> [w246]
              frame #0 {
                # "LAB01-1"
                n165 = Equal?(x=w251, y=2) -> (x = y?=w249:bool)
                n166 = local read "LAB01 (DISP 1)"() -> (w252:T5)
                n167 = Unbundle(w252) -> ("1 (STATUS)"=w253:string)  [unwired: 5 out]
                n168 = Equal?(x=w253, y="RUN") -> (x = y?=w248:bool)
                n169 = And(x=w248, y=w249) -> (x .and. y?=w247:bool)
                n170 = case shown="True" w247 {
                  tunnel: w252 -> [_ w258]
                  tunnel: w246 -> [_ w257]
                  frame False {
                  }
                  frame True {
                    n171 = local read "LAB01 (SETTINGS 1)"() -> (w256:T4)
                    n172 = Unbundle(w258) -> ("1 (CYCLE)"=w259:dbl)  [unwired: 5 out]
                    n173 = Unbundle(w256) -> ("1 (T-RISE mins)"=w255:dbl)  [unwired: 9 out]
                    n174 = Greater Or Equal?(x=w259, y=w257) -> (x >= y?=w260:bool)
                    n175 = case shown="True" w260 {
                      tunnel: w255 -> [w261 _]
                      frame True {
                        n176 = stacked-sequence {
                          tunnel: w261 -> [w263 _]
                          frame #0 {
                            n177 = local read "LAB01-1 (TDMS)"() -> (w268:refnum<k34>)
                            n178 = Build Array("T-RISE") -> (w265:string[])
                            n179 = Build Array(w263) -> (w264:dbl[])
                            n180 = TDMS Write(0:w268, 5:"TEST PASS", 7:w265, 9:w264) -> (15:w267:errorcluster)  [unwired: 2 in, 3 out]
                            n181 = local write "data file error"(w267) -> ()
                          }
                          frame #1 {
                            n182 = local read "LAB01 (DISP 1)"() -> (w271:T5)
                            n183 = Bundle(cluster=w271, "1 (STATUS)"="STOP") -> (w269:T5)  [unwired: 5 in]
                            n184 = local write "LAB01 (DISP 1)"(w269) -> ()
                          }
                        }
                      }
                      frame False {
                      }
                    }
                  }
                }
              }
            }
          }
          frame #5 {
            # "disable functions"
            n185 = stacked-sequence {
              tunnel: w281 -> [w286 _ w341]
              tunnel: w280 -> [w285 _ w340]
              tunnel: w279 -> [w284 _ w339]
              tunnel: w278 -> [w283 _ w338]
              tunnel: w277 -> [w282 _ w337]
              tunnel: w276 -> [_ w306 w336]
              tunnel: w275 -> [_ w305 w335]
              tunnel: w274 -> [_ w304 w334]
              tunnel: w273 -> [_ w303 w333]
              tunnel: w272 -> [_ w302 w332]
              frame #0 {
                n186 = Select(t=2, s=w283, f=0) -> (s? t:f=w290:i32)
                n187 = Select(t=2, s=w284, f=0) -> (s? t:f=w293:i32)
                n188 = Select(t=2, s=w282, f=0) -> (s? t:f=w287:i32)
                n189 = Select(t=2, s=w286, f=0) -> (s? t:f=w299:i32)
                n190 = Select(t=2, s=w285, f=0) -> (s? t:f=w296:i32)
                n191 = property on="LAB02-2 SELECT" class="RadioBtnsControl (strict)"("DisabledEnum"=w290) -> ()  [unwired: 2 in, 2 out]
                n192 = property on="LAB02-1 SELECT" class="RadioBtnsControl (strict)"("DisabledEnum"=w293) -> ()  [unwired: 2 in, 2 out]
                n193 = property on="LAB03-1 SELECT" class="RadioBtnsControl (strict)"("DisabledEnum"=w287) -> ()  [unwired: 2 in, 2 out]
                n194 = property on="LAB01-1 SELECT" class="RadioBtnsControl (strict)"("DisabledEnum"=w299) -> ()  [unwired: 2 in, 2 out]
                n195 = property on="LAB01-2 SELECT" class="RadioBtnsControl (strict)"("DisabledEnum"=w296) -> ()  [unwired: 2 in, 2 out]
              }
              frame #1 {
                n196 = Select(t=2, s=w302, f=0) -> (s? t:f=w307:i32)
                n197 = Select(t=2, s=w303, f=0) -> (s? t:f=w310:i32)
                n198 = Select(t=2, s=w306, f=0) -> (s? t:f=w319:i32)
                n199 = Select(t=2, s=w305, f=0) -> (s? t:f=w316:i32)
                n200 = Select(t=2, s=w304, f=0) -> (s? t:f=w313:i32)
                n201 = property on="LAB05-2 SELECT" class="RadioBtnsControl (strict)"("DisabledEnum"=w307) -> ()  [unwired: 2 in, 2 out]
                n202 = property on="LAB05-1 SELECT" class="RadioBtnsControl (strict)"("DisabledEnum"=w310) -> ()  [unwired: 2 in, 2 out]
                n203 = property on="LAB03-2 SELECT" class="RadioBtnsControl (strict)"("DisabledEnum"=w319) -> ()  [unwired: 2 in, 2 out]
                n204 = property on="LAB04-1 SELECT" class="RadioBtnsControl (strict)"("DisabledEnum"=w316) -> ()  [unwired: 2 in, 2 out]
                n205 = property on="LAB04-2 SELECT" class="RadioBtnsControl (strict)"("DisabledEnum"=w313) -> ()  [unwired: 2 in, 2 out]
              }
              frame #2 {
                # "disable calibrate if any test running"
                n206 = Or(x=w333, y=w332) -> (x .or. y?=w326:bool)
                n207 = Or(x=w335, y=w334) -> (x .or. y?=w328:bool)
                n208 = Or(x=w339, y=w338) -> (x .or. y?=w330:bool)
                n209 = Or(x=w337, y=w336) -> (x .or. y?=w329:bool)
                n210 = Or(x=w341, y=w340) -> (x .or. y?=w331:bool)
                n211 = Or(x=w329, y=w328) -> (x .or. y?=w327:bool)
                n212 = Or(x=w331, y=w330) -> (x .or. y?=w325:bool)
                n213 = Or(x=w327, y=w326) -> (x .or. y?=w324:bool)
                n214 = Or(x=w325, y=w324) -> (x .or. y?=w323:bool)
                n215 = case shown="True" w323 {
                  tunnel: [0 2] -> w322
                  frame False {
                  }
                  frame True {
                  }
                }
                n216 = property on="CALIBRATE" class="Bool (strict)"("DisabledEnum"=w322) -> ()  [unwired: 2 in, 2 out]
              }
            }
          }
          frame #6 {
            # "check for RUN switch change, start test if true and stop test if false"
            n217 = Get Date/Time In Seconds() -> (seconds since 1Jan1904=w348:timestamp)
            n218 = Format Date/Time String(time format string (%c)="%Y%m%d", seconds (now)=w348) -> (date/time string=w349:string)  [unwired: 1 in]
            n219 = Format Date/Time String(time format string (%c)="%H%M", seconds (now)=w348) -> (date/time string=w346:string)  [unwired: 1 in]
            n220 = event shown="[1] \"LAB01-1RUN\": Value Change" {
              selector: _ -> [_ _]
              dyn-events: _ -> [_ _]
              timeout: 10 -> [_ _]
              tunnel: "c:\\crabtree\\Test Data\\" -> [_ w357]
              tunnel: w349 -> [_ w356]
              tunnel: w346 -> [_ w354]
              tunnel: w345 -> [_ w355]
              tunnel: w344 -> [_ w353]
              event Timeout {
                n221 = event-data() -> ()  [unwired: 1 in, 3 out]
              }
              event "LAB01-1RUN": Value Change {
                n222 = event-data() -> ()  [unwired: 1 in, 6 out]
                n223 = case shown="False" w353 {
                  tunnel: w357 -> [_ w379]
                  tunnel: w356 -> [_ w378]
                  tunnel: w355 -> [w358 w377]
                  tunnel: w354 -> [_ w376]
                  tunnel: w353 -> [_ w375]
                  frame False {
                    # "stop test"
                    n224 = stacked-sequence {
                      tunnel: w358 -> [w364 _]
                      frame #0 {
                        n225 = local read "LAB01 (DISP 1)"() -> (w363:T5)
                        n226 = Unbundle(w363) -> ("1 (CYCLE)"=w361:dbl, "1 (T-RISE min)"=w362:dbl)  [unwired: 4 out]
                        n227 = case shown="\"CYCLE TEST\"" w364 {
                          tunnel: w362 -> [_ _ w371]
                          tunnel: w361 -> [w369 w370 _]
                          tunnel: [w369 w370 w371] -> w360
                          frame "TEST SET UP", Default {
                          }
                          frame "CYCLE TEST" {
                          }
                          frame "T-RISE TEST" {
                          }
                        }
                        n228 = local read "LAB01-1 (TDMS)"() -> (w368:refnum<k34>)
                        n229 = Build Array("STOPPED") -> (w365:string[])
                        n230 = Build Array(w360) -> (w359:dbl[])
                        n231 = TDMS Write(0:w368, 5:"TEST RESULT", 7:w365, 9:w359) -> ()  [unwired: 2 in, 4 out]
                      }
                      frame #1 {
                        n232 = local read "LAB01 (DISP 1)"() -> (w374:T5)
                        n233 = Bundle(cluster=w374, "1 (STATUS)"="STOP") -> (w372:T5)  [unwired: 5 in]
                        n234 = local write "LAB01 (DISP 1)"(w372) -> ()
                      }
                    }
                  }
                  frame True {
                    # "start new test and create test file"
                    n235 = stacked-sequence {
                      seq-local: [w385 _ _ _ _] -> [_ w398 _ _ _]
                      tunnel: w379 -> [w394 _ _ _ _]
                      tunnel: w378 -> [w392 _ _ _ _]
                      tunnel: w377 -> [w391 _ _ _ _]
                      tunnel: w376 -> [w382 _ _ _ _]
                      tunnel: w375 -> [_ w399 _ _ _]
                      frame #0 {
                        n236 = local read "LAB01 (SETTINGS 1)"() -> (w384:T4)
                        n237 = case shown="\"TEST SET UP\", Default" w391 {
                          tunnel: ["TEST SET UP-" "CYCLE TEST-" "T-RISE TEST-"] -> w387
                          frame "TEST SET UP", Default {
                          }
                          frame "CYCLE TEST" {
                          }
                          frame "T-RISE TEST" {
                          }
                        }
                        n238 = Unbundle(w384) -> ("1 Description"=w383:string)  [unwired: 9 out]
                        n239 = Concatenate Strings(w394, "LAB01-1\\", w392, "\\") -> (w388:string)
                        n240 = String To Path(string=w388) -> (path=w390:path)
                        n241 = Concatenate Strings(w388, w387, w383, "-", w382, ".tdms") -> (w385:string)
                        n242 = Create Folder(path (use dialog)=w390) -> (error out=w389:errorcluster)  [unwired: 2 in, 2 out]
                        n243 = call <vilib>:"Clear Errors.vi"("error in (no error)"=w389) -> ()  [unwired: 6 in, 1 out]
                      }
                      frame #1 {
                        n244 = case shown="True" w399 {
                          tunnel: w398 -> [_ w400]
                          frame False {
                          }
                          frame True {
                            n245 = String To Path(string=w400) -> (path=w401:path)
                            n246 = TDMS Open(5:FALSE, 6:FALSE, 10:T14."create or replace" ("operation (0:open)"), 11:w401) -> (0:w403:errorcluster, 3:→"LAB01-1 (TDMS)":refnum<k34>)  [unwired: 3 in]
                            n247 = local write "data file error"(w403) -> ()
                          }
                        }
                      }
                      frame #2 {
                        n248 = local read "LAB01 (SETTINGS 1)"() -> (w412:T4)
                        n249 = local read "LAB01-1 (TDMS)"() -> (w423:refnum<k34>)
                        n250 = Build Array("Testers Name", "Description", "Set Test Cycles", "T-Rise minutes", "T-Rise Deg C") -> (w413:string[])
                        n251 = Unbundle(w412) -> ("1 Name"=w411:string, "1 Description"=w410:string, "1 (CYCLES)"=w409:dbl, "1 (T-RISE mins)"=w408:dbl, "1 (T-RISE deg C)"=w407:dbl)  [unwired: 5 out]
                        n252 = Number To Decimal String(number=w409) -> (decimal integer string=w422:string)  [unwired: 1 in]
                        n253 = Number To Decimal String(number=w408) -> (decimal integer string=w421:string)  [unwired: 1 in]
                        n254 = Number To Decimal String(number=w407) -> (decimal integer string=w420:string)  [unwired: 1 in]
                        n255 = Build Array(w411, w410, w422, w421, w420) -> (w419:string[])
                        n256 = TDMS Set Properties(5:w419, 7:w413, 11:w423) -> ()  [unwired: 3 in, 4 out]
                      }
                      frame #3 {
                        w425 = 0.0
                        n257 = local read "LAB01 (DISP 1)"() -> (w427:T5)
                        n258 = Bundle(cluster=w427, "1 (CYCLE)"=w425, "1 (T-RISE min)"=w425, "1 (STATUS)"="RUN") -> (w426:T5)  [unwired: 3 in]
                        n259 = local write "LAB01 (DISP 1)"(w426) -> ()
                      }
                      frame #4 {
                        n260 = local read "LAB01-1 (SIG)"() -> (w430:T2)
                        n261 = local read "LAB01 (TEMP START)"() -> (w432:T6)
                        n262 = Unbundle(w430) -> ("Tmp Live"=w429:dbl, "Tmp Neut"=w428:dbl)  [unwired: 3 out]
                        n263 = Bundle(cluster=w432, "1 (TL)"=w429, "1 (TN)"=w428) -> (w431:T6)  [unwired: 2 in]
                        n264 = local write "LAB01 (TEMP START)"(w431) -> ()
                      }
                    }
                  }
                }
              }
            }
          }
          frame #7 {
            # "end test & close test files"
            n265 = stacked-sequence {
              frame #0 {
                n266 = local read "LAB01 (DISP 1)"() -> (w434:T5)
                n267 = Unbundle(w434) -> ("1 (STATUS)"=w433:string)  [unwired: 5 out]
                n268 = Equal?(x=w433, y="STOP") -> (x = y?=w435:bool)
                n269 = case shown="True" w435 {
                  frame False {
                  }
                  frame True {
                    n270 = stacked-sequence {
                      frame #0 {
                        n271 = local read "LAB01 (DISP 1)"() -> (w439:T5)
                        n272 = Bundle(cluster=w439, "1 (STATUS)"="END") -> (w437:T5)  [unwired: 5 in]
                        n273 = local write "LAB01 (DISP 1)"(w437) -> ()
                      }
                      frame #1 {
                        n274 = local read "LAB01-1 (TDMS)"() -> (w442:refnum<k34>)
                        n275 = TDMS Close(11:w442) -> (0:w441:errorcluster)  [unwired: 1 in, 1 out]
                        n276 = local write "LAB01-1RUN"(FALSE) -> ()
                        n277 = local write "data file error"(w441) -> ()
                      }
                    }
                  }
                }
              }
            }
          }
          frame #8 {
            # "drive jigs"
            n278 = stacked-sequence {
              frame #0 {
                # "jig on"
                n279 = local read "jig cycle"() -> (w443:dbl)
                n280 = Equal?(x=w443, y=0) -> (x = y?=w445:bool)
                n281 = case shown="True" w445 {
                  frame False {
                  }
                  frame True {
                    n282 = local read "LAB01-1RUN"() -> (w446:bool)
                    n283 = local read "LAB01-2 RUN"() -> (w447:bool)
                    n284 = local read "LAB03-1 RUN"() -> (w453:bool)
                    n285 = local read "LAB03-2 RUN"() -> (w452:bool)
                    n286 = local read "LAB02-1 RUN"() -> (w455:bool)
                    n287 = local read "LAB02-2 RUN"() -> (w454:bool)
                    n288 = local read "LAB04-1 RUN"() -> (w451:bool)
                    n289 = local read "LAB04-2 RUN"() -> (w450:bool)
                    n290 = local read "LAB05-1 RUN"() -> (w449:bool)
                    n291 = local read "LAB05-2 RUN"() -> (w448:bool)
                    n292 = local write "LAB05-1 (JIG)"(w449) -> ()
                    n293 = local write "LAB05-2 (JIG)"(w448) -> ()
                    n294 = local write "LAB04-2 (JIG)"(w450) -> ()
                    n295 = local write "LAB02-1 (JIG)"(w455) -> ()
                    n296 = local write "LAB03-1 (JIG)"(w453) -> ()
                    n297 = local write "LAB04-1 (JIG)"(w451) -> ()
                    n298 = local write "LAB03-2 (JIG)"(w452) -> ()
                    n299 = local write "LAB02-2 (JIG)"(w454) -> ()
                    n300 = local write "LAB01-1 (JIG)"(w446) -> ()
                    n301 = local write "LAB01-2 (JIG)"(w447) -> ()
                  }
                }
              }
              frame #1 {
                # "jig off"
                n302 = local read "jig cycle"() -> (w458:dbl)
                n303 = local read "on loops"() -> (w457:dbl)
                n304 = Equal?(x=w458, y=w457) -> (x = y?=w456:bool)
                n305 = case shown="True" w456 {
                  frame False {
                  }
                  frame True {
                    w509 = FALSE
                    w510 = TRUE
                    w508 = 2
                    n306 = local read "LAB05-2 SELECT"() -> (w499:T3)
                    n307 = local read "LAB04-2 SELECT"() -> (w501:T3)
                    n308 = local read "LAB04-1 SELECT"() -> (w502:T3)
                    n309 = local read "LAB05-1 SELECT"() -> (w500:T3)
                    n310 = local read "LAB03-2 SELECT"() -> (w503:T3)
                    n311 = local read "LAB02-1 SELECT"() -> (w506:T3)
                    n312 = local read "LAB03-1 SELECT"() -> (w504:T3)
                    n313 = local read "LAB02-2 SELECT"() -> (w505:T3)
                    n314 = local read "LAB01-2 SELECT"() -> (w507:T3)
                    n315 = local read "LAB05-1 RUN"() -> (w469:bool)
                    n316 = local read "LAB05-2 RUN"() -> (w468:bool)
                    n317 = local read "LAB04-2 RUN"() -> (w470:bool)
                    n318 = local read "LAB04-1 RUN"() -> (w471:bool)
                    n319 = local read "LAB01-2 RUN"() -> (w476:bool)
                    n320 = local read "LAB03-2 RUN"() -> (w472:bool)
                    n321 = local read "LAB01-1RUN"() -> (w487:bool)
                    n322 = local read "LAB01-1 SELECT"() -> (w511:T3)
                    n323 = local read "LAB03-1 RUN"() -> (w473:bool)
                    n324 = local read "LAB02-1 RUN"() -> (w475:bool)
                    n325 = local read "LAB02-2 RUN"() -> (w474:bool)
                    n326 = Equal?(x=w508, y=w504) -> (x = y?=w482:bool)
                    n327 = Equal?(x=w508, y=w503) -> (x = y?=w481:bool)
                    n328 = Equal?(x=w508, y=w502) -> (x = y?=w480:bool)
                    n329 = Equal?(x=w508, y=w501) -> (x = y?=w479:bool)
                    n330 = Equal?(x=w508, y=w500) -> (x = y?=w478:bool)
                    n331 = Equal?(x=w508, y=w499) -> (x = y?=w477:bool)
                    n332 = Equal?(x=w508, y=w511) -> (x = y?=w488:bool)
                    n333 = Equal?(x=w508, y=w506) -> (x = y?=w484:bool)
                    n334 = Equal?(x=w508, y=w505) -> (x = y?=w483:bool)
                    n335 = Equal?(x=w508, y=w507) -> (x = y?=w485:bool)
                    n336 = And(x=w479, y=w470) -> (x .and. y?=w461:bool)
                    n337 = And(x=w482, y=w473) -> (x .and. y?=w464:bool)
                    n338 = And(x=w480, y=w471) -> (x .and. y?=w462:bool)
                    n339 = And(x=w477, y=w468) -> (x .and. y?=w459:bool)
                    n340 = And(x=w483, y=w474) -> (x .and. y?=w465:bool)
                    n341 = And(x=w481, y=w472) -> (x .and. y?=w463:bool)
                    n342 = And(x=w478, y=w469) -> (x .and. y?=w460:bool)
                    n343 = And(x=w485, y=w476) -> (x .and. y?=w467:bool)
                    n344 = And(x=w488, y=w487) -> (x .and. y?=w486:bool)
                    n345 = And(x=w484, y=w475) -> (x .and. y?=w466:bool)
                    n346 = Select(t=w510, s=w486, f=w509) -> (s? t:f=w489:bool)
                    n347 = Select(t=w510, s=w467, f=w509) -> (s? t:f=w490:bool)
                    n348 = Select(t=w510, s=w466, f=w509) -> (s? t:f=w491:bool)
                    n349 = Select(t=w510, s=w465, f=w509) -> (s? t:f=w492:bool)
                    n350 = Select(t=w510, s=w464, f=w509) -> (s? t:f=w493:bool)
                    n351 = Select(t=w510, s=w463, f=w509) -> (s? t:f=w494:bool)
                    n352 = Select(t=w510, s=w462, f=w509) -> (s? t:f=w495:bool)
                    n353 = Select(t=w510, s=w461, f=w509) -> (s? t:f=w496:bool)
                    n354 = Select(t=w510, s=w460, f=w509) -> (s? t:f=w497:bool)
                    n355 = Select(t=w510, s=w459, f=w509) -> (s? t:f=w498:bool)
                    n356 = local write "LAB03-2 (JIG)"(w494) -> ()
                    n357 = local write "LAB02-1 (JIG)"(w491) -> ()
                    n358 = local write "LAB02-2 (JIG)"(w492) -> ()
                    n359 = local write "LAB01-2 (JIG)"(w490) -> ()
                    n360 = local write "LAB03-1 (JIG)"(w493) -> ()
                    n361 = local write "LAB01-1 (JIG)"(w489) -> ()
                    n362 = local write "LAB05-2 (JIG)"(w498) -> ()
                    n363 = local write "LAB04-1 (JIG)"(w495) -> ()
                    n364 = local write "LAB05-1 (JIG)"(w497) -> ()
                    n365 = local write "LAB04-2 (JIG)"(w496) -> ()
                  }
                }
              }
            }
          }
          frame #9 {
            # "drive digital output"
            n366 = local read "LAB05-2 (O/I)"() -> (w517:bool)
            n367 = local read "LAB05-2 (JIG)"() -> (w516:bool)
            n368 = local read "LAB05-1 (O/I)"() -> (w519:bool)
            n369 = local read "LAB05-1 (JIG)"() -> (w518:bool)
            n370 = local read "LAB04-2 (O/I)"() -> (w521:bool)
            n371 = local read "LAB04-2 (JIG)"() -> (w520:bool)
            n372 = local read "LAB03-1 (O/I)"() -> (w526:bool)
            n373 = local read "LAB04-1 (O/I)"() -> (w522:bool)
            n374 = local read "LAB04-1 (JIG)"() -> (w515:bool)
            n375 = local read "LAB02-1 (O/I)"() -> (w530:bool)
            n376 = local read "LAB02-2 (O/I)"() -> (w528:bool)
            n377 = local read "LAB03-2 (O/I)"() -> (w524:bool)
            n378 = local read "LAB03-2 (JIG)"() -> (w523:bool)
            n379 = local read "LAB02-1 (JIG)"() -> (w529:bool)
            n380 = local read "LAB02-2 (JIG)"() -> (w527:bool)
            n381 = local read "LAB03-1 (JIG)"() -> (w525:bool)
            n382 = local read "LAB01-2 (O/I)"() -> (w532:bool)
            n383 = local read "LAB01-2 (JIG)"() -> (w531:bool)
            n384 = local read "LAB01-1 (O/I)"() -> (w534:bool)
            n385 = local read "LAB01-1 (JIG)"() -> (w533:bool)
            n386 = Build Array(w521, w520, w519, w518, w517, w516) -> (w512:bool[])
            n387 = Build Array(w527, w526, w525, w524, w523, w522, w515) -> (w513:bool[])
            n388 = Build Array(w534, w533, w532, w531, w530, w529, w528) -> (w514:bool[])
            n389 = call "sub vi - Drive Relays All v6.vi"("Array #2"=w512, "Array #1"=w513, "Array #0"=w514) -> ()  [unwired: 8 in, 1 out]
          }
          frame #10 {
            # "get temperature values"
            n390 = stacked-sequence {
              frame #0 {
                n391 = local read "jig cycle"() -> (w535:dbl)
                n392 = local read "on loops"() -> (w538:dbl)
                n393 = local read "jig cycle"() -> (w540:dbl)
                n394 = Add(x=w538, y=1) -> (x+y=w539:dbl)
                n395 = Equal?(x=w540, y=0) -> (x = y?=w541:bool)
                n396 = Equal?(x=w535, y=w539) -> (x = y?=w536:bool)
                n397 = case shown="True" w541 {
                  frame False {
                  }
                  frame True {
                    w553 = FALSE
                    w554 = TRUE
                    n398 = local write "TEMP update"(TRUE) -> ()
                    n399 = call "sub vi - GET ALL TEMP v3.vi"("LA01-EN"=w554, "LA02-EN"=w554, "LA03-EN"=w554, "LA04-EN"=w553, "LA05-EN"=w553, "Gen Cal Value"=1.0) -> ("LA01 TEMP"=w552:T15, "LA02 TEMP"=w550:T15, "LA03 TEMP"=w549:T15)  [unwired: 4 in, 3 out]
                    n400 = local write "LAB03 TEMP"(w549) -> ()
                    n401 = local write "LAB02 TEMP"(w550) -> ()
                    n402 = local write "LAB01 TEMP"(w552) -> ()
                  }
                }
                n403 = case shown="True" w536 {
                  frame False {
                  }
                  frame True {
                    w546 = TRUE
                    w547 = FALSE
                    n404 = local write "TEMP update"(TRUE) -> ()
                    n405 = call "sub vi - GET ALL TEMP v3.vi"("LA01-EN"=w547, "LA02-EN"=w547, "LA03-EN"=w547, "LA04-EN"=w546, "LA05-EN"=w546, "Gen Cal Value"=1.0) -> ("LA04 TEMP"=w544:T15, "LA05 TEMP"=w543:T15)  [unwired: 4 in, 4 out]
                    n406 = local write "LAB04 TEMP"(w544) -> ()
                    n407 = local write "LAB05 TEMP"(w543) -> ()
                  }
                }
              }
              frame #1 {
                n408 = local read "LAB01 (CAL)"() -> (w572:T7)
                n409 = local read "LAB01 TEMP"() -> (w573:T10)
                n410 = Unbundle By Name(w573) -> ("T1 Live"=w563:dbl, "T1 Neut"=w562:dbl, "T2 Live"=w561:dbl, "T2 Neut"=w560:dbl)  [unwired: 2 out]
                n411 = Unbundle By Name(w572) -> ("1 (TL) cal"=w559:dbl, "1 (TN) cal"=w558:dbl, "2 (TL) cal"=w557:dbl, "2 (TN) cal"=w556:dbl)  [unwired: 6 out]
                n412 = Multiply(x=w563, y=w559) -> (x*y=w569:dbl)
                n413 = Multiply(x=w562, y=w558) -> (x*y=w568:dbl)
                n414 = Multiply(x=w561, y=w557) -> (x*y=w565:dbl)
                n415 = Multiply(x=w560, y=w556) -> (x*y=w564:dbl)
                n416 = local read "LAB01-2 (SIG)"() -> (w567:T2)
                n417 = local read "LAB01-1 (SIG)"() -> (w571:T2)
                n418 = Bundle By Name(cluster=w571, "Tmp Live"=w569, "Tmp Neut"=w568) -> (w570:T2)
                n419 = Bundle By Name(cluster=w567, "Tmp Live"=w565, "Tmp Neut"=w564) -> (w566:T2)
                n420 = local write "LAB01-1 (SIG)"(w570) -> ()
                n421 = local write "LAB01-2 (SIG)"(w566) -> ()
              }
              frame #2 {
                n422 = local read "LAB02 (CAL)"() -> (w590:T8)
                n423 = local read "LAB02 TEMP"() -> (w591:T10)
                n424 = Unbundle By Name(w591) -> ("T1 Live"=w581:dbl, "T1 Neut"=w580:dbl, "T2 Live"=w579:dbl, "T2 Neut"=w578:dbl)  [unwired: 2 out]
                n425 = Unbundle By Name(w590) -> ("1 (TL) cal"=w577:dbl, "1 (TN) cal"=w576:dbl, "2 (TL) cal"=w575:dbl, "2 (TN) cal"=w574:dbl)  [unwired: 6 out]
                n426 = Multiply(x=w581, y=w577) -> (x*y=w587:dbl)
                n427 = Multiply(x=w580, y=w576) -> (x*y=w586:dbl)
                n428 = Multiply(x=w579, y=w575) -> (x*y=w583:dbl)
                n429 = Multiply(x=w578, y=w574) -> (x*y=w582:dbl)
                n430 = local read "LAB02-2 (SIG)"() -> (w585:T2)
                n431 = local read "LAB02-1 (SIG)"() -> (w589:T2)
                n432 = Bundle By Name(cluster=w589, "Tmp Live"=w587, "Tmp Neut"=w586) -> (w588:T2)
                n433 = Bundle By Name(cluster=w585, "Tmp Live"=w583, "Tmp Neut"=w582) -> (w584:T2)
                n434 = local write "LAB02-1 (SIG)"(w588) -> ()
                n435 = local write "LAB02-2 (SIG)"(w584) -> ()
              }
              frame #3 {
                n436 = local read "LAB03 (CAL)"() -> (w608:T7)
                n437 = local read "LAB03 TEMP"() -> (w609:T10)
                n438 = Unbundle By Name(w609) -> ("T1 Live"=w599:dbl, "T1 Neut"=w598:dbl, "T2 Live"=w597:dbl, "T2 Neut"=w596:dbl)  [unwired: 2 out]
                n439 = Unbundle By Name(w608) -> ("1 (TL) cal"=w595:dbl, "1 (TN) cal"=w594:dbl, "2 (TL) cal"=w593:dbl, "2 (TN) cal"=w592:dbl)  [unwired: 6 out]
                n440 = Multiply(x=w599, y=w595) -> (x*y=w605:dbl)
                n441 = Multiply(x=w598, y=w594) -> (x*y=w604:dbl)
                n442 = Multiply(x=w597, y=w593) -> (x*y=w601:dbl)
                n443 = Multiply(x=w596, y=w592) -> (x*y=w600:dbl)
                n444 = local read "LAB03-2 (SIG)"() -> (w603:T2)
                n445 = local read "LAB03-1 (SIG)"() -> (w607:T2)
                n446 = Bundle By Name(cluster=w607, "Tmp Live"=w605, "Tmp Neut"=w604) -> (w606:T2)
                n447 = Bundle By Name(cluster=w603, "Tmp Live"=w601, "Tmp Neut"=w600) -> (w602:T2)
                n448 = local write "LAB03-1 (SIG)"(w606) -> ()
                n449 = local write "LAB03-2 (SIG)"(w602) -> ()
              }
              frame #4 {
                n450 = local read "LAB04 (CAL)"() -> (w626:T7)
                n451 = local read "LAB04 TEMP"() -> (w627:T10)
                n452 = Unbundle By Name(w627) -> ("T1 Live"=w617:dbl, "T1 Neut"=w616:dbl, "T2 Live"=w615:dbl, "T2 Neut"=w614:dbl)  [unwired: 2 out]
                n453 = Unbundle By Name(w626) -> ("1 (TL) cal"=w613:dbl, "1 (TN) cal"=w612:dbl, "2 (TL) cal"=w611:dbl, "2 (TN) cal"=w610:dbl)  [unwired: 6 out]
                n454 = Multiply(x=w617, y=w613) -> (x*y=w623:dbl)
                n455 = Multiply(x=w616, y=w612) -> (x*y=w622:dbl)
                n456 = Multiply(x=w615, y=w611) -> (x*y=w619:dbl)
                n457 = Multiply(x=w614, y=w610) -> (x*y=w618:dbl)
                n458 = local read "LAB04-2 (SIG)"() -> (w621:T2)
                n459 = local read "LAB04-1 (SIG)"() -> (w625:T2)
                n460 = Bundle By Name(cluster=w625, "Tmp Live"=w623, "Tmp Neut"=w622) -> (w624:T2)
                n461 = Bundle By Name(cluster=w621, "Tmp Live"=w619, "Tmp Neut"=w618) -> (w620:T2)
                n462 = local write "LAB04-1 (SIG)"(w624) -> ()
                n463 = local write "LAB04-2 (SIG)"(w620) -> ()
              }
              frame #5 {
                n464 = local read "LAB05 (CAL)"() -> (w644:T7)
                n465 = local read "LAB05 TEMP"() -> (w645:T10)
                n466 = Unbundle By Name(w645) -> ("T1 Live"=w635:dbl, "T1 Neut"=w634:dbl, "T2 Live"=w633:dbl, "T2 Neut"=w632:dbl)  [unwired: 2 out]
                n467 = Unbundle By Name(w644) -> ("1 (TL) cal"=w631:dbl, "1 (TN) cal"=w630:dbl, "2 (TL) cal"=w629:dbl, "2 (TN) cal"=w628:dbl)  [unwired: 6 out]
                n468 = Multiply(x=w635, y=w631) -> (x*y=w641:dbl)
                n469 = Multiply(x=w634, y=w630) -> (x*y=w640:dbl)
                n470 = Multiply(x=w633, y=w629) -> (x*y=w637:dbl)
                n471 = Multiply(x=w632, y=w628) -> (x*y=w636:dbl)
                n472 = local read "LAB05-2 (SIG)"() -> (w639:T2)
                n473 = local read "LAB05-1 (SIG)"() -> (w643:T2)
                n474 = Bundle By Name(cluster=w643, "Tmp Live"=w641, "Tmp Neut"=w640) -> (w642:T2)
                n475 = Bundle By Name(cluster=w639, "Tmp Live"=w637, "Tmp Neut"=w636) -> (w638:T2)
                n476 = local write "LAB05-1 (SIG)"(w642) -> ()
                n477 = local write "LAB05-2 (SIG)"(w638) -> ()
              }
            }
          }
          frame #11 {
            # "get analog values"
            n478 = local read "on loops"() -> (w652:dbl)
            n479 = local read "jig cycle"() -> (w649:dbl)
            n480 = Add(x=w652, y=2) -> (x+y=w650:dbl)
            n481 = Equal?(x=w649, y=1) -> (x = y?=w647:bool)
            n482 = Equal?(x=w649, y=w650) -> (x = y?=w648:bool)
            n483 = Or(x=w647, y=w648) -> (x .or. y?=w646:bool)
            n484 = case shown="True" w646 {
              frame False {
              }
              frame True {
                n485 = call "sub vi - Read Analog All v7.vi"() -> ("Analog loop time"=w660:dbl, "array GRAPH"=w659:dynamicdata[], "LAB01"=w658:T16, "LAB02"=w657:T17, "LAB03"=w656:T18, "LAB04"=w655:T19, "array ERROR"=w661:errorcluster[], "LAB05"=w654:T20)  [unwired: 8 in]
                n486 = stacked-sequence {
                  tunnel: w661 -> [w664 _ _ _ _ _]
                  tunnel: w660 -> [w663 _ _ _ _ _]
                  tunnel: w659 -> [w662 _ _ _ _ _]
                  tunnel: w658 -> [_ w709 _ _ _ _]
                  tunnel: w657 -> [_ _ w710 _ _ _]
                  tunnel: w656 -> [_ _ _ w734 _ _]
                  tunnel: w655 -> [_ _ _ _ w758 _]
                  tunnel: w654 -> [_ _ _ _ _ w782]
                  frame #0 {
                    n487 = local write "AI update"(TRUE) -> ()
                    n488 = Index Array(array=w662, index=6) -> (element=→"LAB04-1 (GRAPH)":dynamicdata)
                    n489 = Index Array(array=w662, index=7) -> (element=→"LAB04-2 (GRAPH)":dynamicdata)
                    n490 = Index Array(array=w662, index=9) -> (element=→"LAB05-2 (GRAPH)":dynamicdata)
                    n491 = Index Array(array=w662, index=8) -> (element=→"LAB05-1 (GRAPH)":dynamicdata)
                    n492 = Index Array(array=w662, index=5) -> (element=→"LAB03-2 (GRAPH)":dynamicdata)
                    n493 = Index Array(array=w662, index=0) -> (element=→"LAB01-1 (GRAPH)":dynamicdata)
                    n494 = Index Array(array=w662, index=1) -> (element=→"LAB01-2 (GRAPH)":dynamicdata)
                    n495 = Index Array(array=w662, index=2) -> (element=→"LAB02-1 (GRAPH)":dynamicdata)
                    n496 = Index Array(array=w662, index=3) -> (element=→"LAB02-2 (GRAPH)":dynamicdata)
                    n497 = Index Array(array=w662, index=4) -> (element=→"LAB03-1 (GRAPH)":dynamicdata)
                    "AI loop time" <- w663
                    "Analog Error Array" <- w664
                  }
                  frame #1 {
                    n498 = local read "LAB01 (CAL)"() -> (w708:T7)
                    n499 = Unbundle By Name(w709) -> ("LAB01-1 (A)"=w707:dbl, "LAB01-1 (V)"=w706:dbl, "LAB01-1 (PF)"=w705:dbl, "LAB01-2 (A)"=w704:dbl, "LAB01-2 (V)"=w703:dbl, "LAB01-2 (PF)"=w702:dbl)
                    n500 = Unbundle By Name(w708) -> ("1  (A) cal"=w701:dbl, "1 (V) cal"=w700:dbl, "1 (PF) cal"=w699:dbl, "2 (A) cal"=w698:dbl, "2 (V) cal"=w697:dbl, "2 (PF) cal"=w696:dbl)  [unwired: 4 out]
                    n501 = Multiply(x=w707, y=w701) -> (x*y=w694:dbl)
                    n502 = Multiply(x=w706, y=w700) -> (x*y=w693:dbl)
                    n503 = Multiply(x=w705, y=w699) -> (x*y=w692:dbl)
                    n504 = Multiply(x=w704, y=w698) -> (x*y=w688:dbl)
                    n505 = local read "LAB01-1 (SIG)"() -> (w695:T2)
                    n506 = Multiply(x=w703, y=w697) -> (x*y=w687:dbl)
                    n507 = Multiply(x=w702, y=w696) -> (x*y=w686:dbl)
                    n508 = local read "LAB01-2 (SIG)"() -> (w690:T2)
                    n509 = Bundle By Name(cluster=w695, "AMPS"=w694, "VOLTS"=w693, "PF"=w692) -> (w691:T2)
                    n510 = Bundle By Name(cluster=w690, "AMPS"=w688, "VOLTS"=w687, "PF"=w686) -> (w689:T2)
                    n511 = local write "LAB01-2 (SIG)"(w689) -> ()
                    n512 = local write "LAB01-1 (SIG)"(w691) -> ()
                  }
                  frame #2 {
                    n513 = local read "LAB02 (CAL)"() -> (w733:T8)
                    n514 = Unbundle By Name(w710) -> ("LAB02-1 (A)"=w732:dbl, "LAB02-1 (V)"=w731:dbl, "LAB02-1 (PF)"=w730:dbl, "LAB02-2 (A)"=w729:dbl, "LAB02-2 (V)"=w728:dbl, "LAB02-2 (PF)"=w727:dbl)
                    n515 = Unbundle By Name(w733) -> ("1 (A) cal"=w726:dbl, "1 (V) cal"=w725:dbl, "1 (PF) cal"=w724:dbl, "2 (A) cal"=w723:dbl, "2 (V) cal"=w722:dbl, "2 (PF) cal"=w721:dbl)  [unwired: 4 out]
                    n516 = Multiply(x=w732, y=w726) -> (x*y=w719:dbl)
                    n517 = Multiply(x=w731, y=w725) -> (x*y=w718:dbl)
                    n518 = Multiply(x=w730, y=w724) -> (x*y=w717:dbl)
                    n519 = Multiply(x=w729, y=w723) -> (x*y=w713:dbl)
                    n520 = local read "LAB02-1 (SIG)"() -> (w720:T2)
                    n521 = Multiply(x=w728, y=w722) -> (x*y=w712:dbl)
                    n522 = Multiply(x=w727, y=w721) -> (x*y=w711:dbl)
                    n523 = local read "LAB02-2 (SIG)"() -> (w715:T2)
                    n524 = Bundle By Name(cluster=w720, "AMPS"=w719, "VOLTS"=w718, "PF"=w717) -> (w716:T2)
                    n525 = Bundle By Name(cluster=w715, "AMPS"=w713, "VOLTS"=w712, "PF"=w711) -> (w714:T2)
                    n526 = local write "LAB02-2 (SIG)"(w714) -> ()
                    n527 = local write "LAB02-1 (SIG)"(w716) -> ()
                  }
                  frame #3 {
                    n528 = local read "LAB03 (CAL)"() -> (w757:T7)
                    n529 = Unbundle By Name(w734) -> ("LAB03-1 (A)"=w756:dbl, "LAB03-1 (V)"=w755:dbl, "LAB03-1 (PF)"=w754:dbl, "LAB03-2 (A)"=w753:dbl, "LAB03-2 (V)"=w752:dbl, "LAB03-2 (PF)"=w751:dbl)
                    n530 = Unbundle By Name(w757) -> ("1  (A) cal"=w750:dbl, "1 (V) cal"=w749:dbl, "1 (PF) cal"=w748:dbl, "2 (A) cal"=w747:dbl, "2 (V) cal"=w746:dbl, "2 (PF) cal"=w745:dbl)  [unwired: 4 out]
                    n531 = Multiply(x=w756, y=w750) -> (x*y=w743:dbl)
                    n532 = Multiply(x=w755, y=w749) -> (x*y=w742:dbl)
                    n533 = Multiply(x=w754, y=w748) -> (x*y=w741:dbl)
                    n534 = Multiply(x=w753, y=w747) -> (x*y=w737:dbl)
                    n535 = local read "LAB03-1 (SIG)"() -> (w744:T2)
                    n536 = Multiply(x=w752, y=w746) -> (x*y=w736:dbl)
                    n537 = Multiply(x=w751, y=w745) -> (x*y=w735:dbl)
                    n538 = local read "LAB03-1 (SIG)"() -> (w739:T2)
                    n539 = Bundle By Name(cluster=w744, "AMPS"=w743, "VOLTS"=w742, "PF"=w741) -> (w740:T2)
                    n540 = Bundle By Name(cluster=w739, "AMPS"=w737, "VOLTS"=w736, "PF"=w735) -> (w738:T2)
                    n541 = local write "LAB03-1 (SIG)"(w738) -> ()
                    n542 = local write "LAB03-1 (SIG)"(w740) -> ()
                  }
                  frame #4 {
                    n543 = local read "LAB04 (CAL)"() -> (w781:T7)
                    n544 = Unbundle By Name(w758) -> ("LAB04-1 (A)"=w780:dbl, "LAB04-1 (V)"=w779:dbl, "LAB04-1 (PF)"=w778:dbl, "LAB04-2 (A)"=w777:dbl, "LAB04-2 (V)"=w776:dbl, "LAB04-2 (PF)"=w775:dbl)
                    n545 = Unbundle By Name(w781) -> ("1  (A) cal"=w774:dbl, "1 (V) cal"=w773:dbl, "1 (PF) cal"=w772:dbl, "2 (A) cal"=w771:dbl, "2 (V) cal"=w770:dbl, "2 (PF) cal"=w769:dbl)  [unwired: 4 out]
                    n546 = Multiply(x=w780, y=w774) -> (x*y=w767:dbl)
                    n547 = Multiply(x=w779, y=w773) -> (x*y=w766:dbl)
                    n548 = Multiply(x=w778, y=w772) -> (x*y=w765:dbl)
                    n549 = Multiply(x=w777, y=w771) -> (x*y=w761:dbl)
                    n550 = local read "LAB04-1 (SIG)"() -> (w768:T2)
                    n551 = Multiply(x=w776, y=w770) -> (x*y=w760:dbl)
                    n552 = Multiply(x=w775, y=w769) -> (x*y=w759:dbl)
                    n553 = local read "LAB04-2 (SIG)"() -> (w763:T2)
                    n554 = Bundle By Name(cluster=w768, "AMPS"=w767, "VOLTS"=w766, "PF"=w765) -> (w764:T2)
                    n555 = Bundle By Name(cluster=w763, "AMPS"=w761, "VOLTS"=w760, "PF"=w759) -> (w762:T2)
                    n556 = local write "LAB04-2 (SIG)"(w762) -> ()
                    n557 = local write "LAB04-1 (SIG)"(w764) -> ()
                  }
                  frame #5 {
                    n558 = local read "LAB05 (CAL)"() -> (w805:T7)
                    n559 = Unbundle By Name(w782) -> ("LAB05-1 (A)"=w804:dbl, "LAB05-1 (V)"=w803:dbl, "LAB05-1 (PF)"=w802:dbl, "LAB05-2 (A)"=w801:dbl, "LAB05-2 (V)"=w800:dbl, "LAB05-2 (PF)"=w799:dbl)
                    n560 = Unbundle By Name(w805) -> ("1  (A) cal"=w798:dbl, "1 (V) cal"=w797:dbl, "1 (PF) cal"=w796:dbl, "2 (A) cal"=w795:dbl, "2 (V) cal"=w794:dbl, "2 (PF) cal"=w793:dbl)  [unwired: 4 out]
                    n561 = Multiply(x=w804, y=w798) -> (x*y=w791:dbl)
                    n562 = Multiply(x=w803, y=w797) -> (x*y=w790:dbl)
                    n563 = Multiply(x=w802, y=w796) -> (x*y=w789:dbl)
                    n564 = Multiply(x=w801, y=w795) -> (x*y=w785:dbl)
                    n565 = local read "LAB05-1 (SIG)"() -> (w792:T2)
                    n566 = Multiply(x=w800, y=w794) -> (x*y=w784:dbl)
                    n567 = Multiply(x=w799, y=w793) -> (x*y=w783:dbl)
                    n568 = local read "LAB05-2 (SIG)"() -> (w787:T2)
                    n569 = Bundle By Name(cluster=w792, "AMPS"=w791, "VOLTS"=w790, "PF"=w789) -> (w788:T2)
                    n570 = Bundle By Name(cluster=w787, "AMPS"=w785, "VOLTS"=w784, "PF"=w783) -> (w786:T2)
                    n571 = local write "LAB05-2 (SIG)"(w786) -> ()
                    n572 = local write "LAB05-1 (SIG)"(w788) -> ()
                  }
                }
              }
            }
          }
          frame #12 {
            # "save test data to file"
            n573 = local read "on loops"() -> (w813:dbl)
            n574 = local read "jig cycle"() -> (w810:dbl)
            n575 = Add(x=w813, y=2) -> (x+y=w811:dbl)
            n576 = Equal?(x=w810, y=1) -> (x = y?=w808:bool)
            n577 = Equal?(x=w810, y=w811) -> (x = y?=w809:bool)
            n578 = Or(x=w808, y=w809) -> (x .or. y?=w807:bool)
            n579 = case shown="True" w807 {
              tunnel: w806 -> [_ w815]
              frame False {
              }
              frame True {
                n580 = stacked-sequence {
                  tunnel: w815 -> [w816]
                  frame #0 {
                    # "LAB01-1"
                    n581 = case shown="True" w816 {
                      frame False {
                      }
                      frame True {
                        n582 = local read "LAB01 (DISP 1)"() -> (w858:T5)
                        n583 = local read "LAB01-1 (SIG)"() -> (w859:T2)
                        n584 = local read "LAB01-1 (TDMS)"() -> (w860:refnum<k34>)
                        n585 = Build Array("TEMP Neut") -> (w824:string[])
                        n586 = Build Array("CYCLE") -> (w819:string[])
                        n587 = Build Array("TEMP Live") -> (w829:string[])
                        n588 = Build Array("PF") -> (w834:string[])
                        n589 = Build Array("AMPS") -> (w855:string[])
                        n590 = Build Array("VOLTS") -> (w846:string[])
                        n591 = Unbundle(w859) -> ("AMPS"=w854:dbl, "VOLTS"=w843:dbl, "PF"=w842:dbl, "Tmp Live"=w841:dbl, "Tmp Neut"=w844:dbl)
                        n592 = Unbundle(w858) -> ("1 (CYCLE)"=w839:dbl)  [unwired: 5 out]
                        n593 = Build Array(w843) -> (w840:dbl[])
                        n594 = Build Array(w842) -> (w833:dbl[])
                        n595 = Build Array(w841) -> (w828:dbl[])
                        n596 = Build Array(w844) -> (w823:dbl[])
                        n597 = Build Array(w854) -> (w853:dbl[])
                        n598 = Build Array(w839) -> (w818:dbl[])
                        n599 = TDMS Write(0:w860, 5:"LAB01-1 TEST VALUES", 7:w855, 9:w853) -> (4:w848:refnum<k34>, 6:w847:string, 15:w835:errorcluster)  [unwired: 2 in, 1 out]
                        n600 = TDMS Write(0:w848, 5:w847, 7:w846, 9:w840, 11:w835) -> (4:w838:refnum<k34>, 6:w837:string, 15:w836:errorcluster)  [unwired: 1 in, 1 out]
                        n601 = TDMS Write(0:w838, 5:w837, 7:w834, 9:w833, 11:w836) -> (4:w832:refnum<k34>, 6:w831:string, 15:w830:errorcluster)  [unwired: 1 in, 1 out]
                        n602 = TDMS Write(0:w832, 5:w831, 7:w829, 9:w828, 11:w830) -> (4:w827:refnum<k34>, 6:w826:string, 15:w825:errorcluster)  [unwired: 1 in, 1 out]
                        n603 = TDMS Write(0:w827, 5:w826, 7:w824, 9:w823, 11:w825) -> (4:w822:refnum<k34>, 6:w821:string, 15:w820:errorcluster)  [unwired: 1 in, 1 out]
                        n604 = TDMS Write(0:w822, 5:w821, 7:w819, 9:w818, 11:w820) -> (15:w817:errorcluster)  [unwired: 1 in, 3 out]
                        n605 = local write "data file error"(w817) -> ()
                      }
                    }
                  }
                }
              }
            }
          }
          frame #13 {
            # "check for cycle test fail conditions"
            n606 = local read "on loops"() -> (w868:dbl)
            n607 = local read "jig cycle"() -> (w865:dbl)
            n608 = local read "jig cycle"() -> (w870:dbl)
            n609 = Add(x=w868, y=2.0) -> (x+y=w866:dbl)
            n610 = Equal?(x=w870, y=1.0) -> (x = y?=w863:bool)
            n611 = Equal?(x=w865, y=w866) -> (x = y?=w861:bool)
            n612 = stacked-sequence {
              tunnel: w864 -> [w880]
              tunnel: w863 -> [w872]
              tunnel: w862 -> [w879]
              tunnel: w861 -> [w871]
              frame #0 {
                # "LAB01-1"
                n613 = case shown="\"T-RISE TEST\"" w880 {
                  tunnel: [FALSE TRUE FALSE] -> w878
                  frame "TEST SET UP", Default {
                  }
                  frame "CYCLE TEST" {
                  }
                  frame "T-RISE TEST" {
                  }
                }
                n614 = Or(x=w872, y=w871) -> (x .or. y?=w876:bool)
                n615 = local read "LAB01-1 (SIG)"() -> (w874:T2)
                n616 = And(x=w879, y=w876) -> (x .and. y?=w875:bool)
                n617 = Unbundle(w874) -> ("AMPS"=w873:dbl)  [unwired: 4 out]
                n618 = And(x=w878, y=w875) -> (x .and. y?=w877:bool)
                n619 = stacked-sequence {
                  tunnel: w877 -> [w887]
                  tunnel: w873 -> [w886]
                  tunnel: w872 -> [w885]
                  tunnel: w871 -> [w884]
                  frame #0 {
                    n620 = case shown="True" w887 {
                      tunnel: w886 -> [_ w893]
                      tunnel: w885 -> [_ w895]
                      tunnel: w884 -> [_ w894]
                      frame False {
                      }
                      frame True {
                        # "check for amps fail"
                        n621 = case shown="True" w894 {
                          tunnel: w893 -> [_ w900]
                          tunnel: [FALSE w899] -> w891
                          tunnel: ["" "AMPS HI"] -> w889
                          frame False {
                          }
                          frame True {
                            n622 = Greater?(x=w900, y=5.0) -> (0:w899:bool)
                          }
                        }
                        n623 = case shown="True" w895 {
                          tunnel: w893 -> [_ w906]
                          tunnel: [FALSE w905] -> w892
                          tunnel: ["" "AMPS LO"] -> w888
                          frame False {
                          }
                          frame True {
                            n624 = Less?(x=w906, y=5.0) -> (x < y?=w905:bool)
                          }
                        }
                        n625 = Or(x=w892, y=w891) -> (x .or. y?=w890:bool)
                        n626 = case shown="True" w890 {
                          tunnel: w889 -> [_ w909]
                          tunnel: w888 -> [_ w908]
                          frame False {
                          }
                          frame True {
                            n627 = stacked-sequence {
                              tunnel: w909 -> [w913 _]
                              tunnel: w908 -> [w912 _]
                              frame #0 {
                                n628 = local read "LAB01-1 (TDMS)"() -> (w916:refnum<k34>)
                                n629 = Build Array(w913, w912) -> (w911:string[])
                                n630 = TDMS Write(0:w916, 5:"TEST RESULT", 7:"AMPS FAIL ", 9:w911) -> (15:w915:errorcluster)  [unwired: 2 in, 3 out]
                                n631 = local write "data file error"(w915) -> ()
                              }
                              frame #1 {
                                n632 = local read "LAB01 (DISP 1)"() -> (w919:T5)
                                n633 = Bundle(cluster=w919, "1 (STATUS)"="STOP") -> (w918:T5)  [unwired: 5 in]
                                n634 = local write "LAB01 (DISP 1)"(w918) -> ()
                              }
                            }
                          }
                        }
                      }
                    }
                  }
                }
              }
            }
          }
          frame #14 {
            # "check for temperature rise test fail conditions"
            n635 = stacked-sequence {
              tunnel: w921 -> [w941]
              tunnel: w920 -> [w940]
              frame #0 {
                # "LAB01-1"
                n636 = local read "LAB01 (DISP 1)"() -> (w925:T5)
                n637 = local read "LAB01 (TEMP START)"() -> (w934:T6)
                n638 = local read "LAB01 (SETTINGS 1)"() -> (w929:T4)
                n639 = local read "LAB01-1 (SIG)"() -> (w936:T2)
                n640 = case shown="\"T-RISE TEST\"" w941 {
                  tunnel: [FALSE FALSE TRUE] -> w939
                  frame "TEST SET UP", Default {
                  }
                  frame "CYCLE TEST" {
                  }
                  frame "T-RISE TEST" {
                  }
                }
                n641 = Unbundle(w929) -> ("1 (T-RISE deg C)"=w926:dbl)  [unwired: 9 out]
                n642 = Unbundle(w934) -> ("1 (TL)"=w931:dbl, "1 (TN)"=w930:dbl)  [unwired: 2 out]
                n643 = Unbundle(w925) -> ("1 (CYCLE)"=w924:dbl)  [unwired: 5 out]
                n644 = Unbundle(w936) -> ("AMPS"=w935:dbl, "Tmp Live"=w933:dbl, "Tmp Neut"=w932:dbl)  [unwired: 2 out]
                n645 = Subtract(x=w933, y=w931) -> (x-y=w928:dbl)
                n646 = Greater?(x=w924, y=2.0) -> (0:w923:bool)
                n647 = Subtract(x=w932, y=w930) -> (x-y=w927:dbl)
                n648 = And(x=w940, y=w923) -> (x .and. y?=w937:bool)
                n649 = And(x=w939, y=w937) -> (x .and. y?=w938:bool)
                n650 = case shown="True" w938 {
                  tunnel: w935 -> [_ w957]
                  tunnel: w928 -> [_ w950]
                  tunnel: w927 -> [_ w949]
                  tunnel: w926 -> [_ w948]
                  frame False {
                  }
                  frame True {
                    # "check for amps & t-rise fail"
                    n651 = Less?(x=w957, y=5.0) -> (x < y?=w943:bool)
                    n652 = Greater?(x=w950, y=w948) -> (0:w953:bool)
                    n653 = Greater?(x=w949, y=w948) -> (0:w954:bool)
                    n654 = Or(x=w953, y=w954) -> (x .or. y?=w942:bool)
                    n655 = Select(t="AMPS LO", s=w943, f="") -> (s? t:f=w944:string)
                    n656 = Select(t="T-RISE HI", s=w942, f="") -> (s? t:f=w945:string)
                    n657 = Or(x=w943, y=w942) -> (x .or. y?=w956:bool)
                    n658 = case shown="True" w956 {
                      tunnel: w945 -> [_ w959]
                      tunnel: w944 -> [_ w958]
                      frame False {
                      }
                      frame True {
                        n659 = stacked-sequence {
                          tunnel: w959 -> [w961 _]
                          tunnel: w958 -> [w960 _]
                          frame #0 {
                            n660 = local read "LAB01-1 (TDMS)"() -> (w966:refnum<k34>)
                            n661 = Build Array(w960, w961) -> (w963:string[])
                            n662 = TDMS Write(0:w966, 5:"TEST RESULT", 7:"T-RISE FAIL ", 9:w963) -> (15:w965:errorcluster)  [unwired: 2 in, 3 out]
                            n663 = local write "data file error"(w965) -> ()
                          }
                          frame #1 {
                            n664 = local read "LAB01 (DISP 1)"() -> (w969:T5)
                            n665 = Bundle(cluster=w969, "1 (STATUS)"="STOP") -> (w968:T5)  [unwired: 5 in]
                            n666 = local write "LAB01 (DISP 1)"(w968) -> ()
                          }
                        }
                      }
                    }
                  }
                }
              }
            }
          }
          frame #15 {
            # "run calibration routine"
            n667 = local read "CALIBRATE"() -> (w973:bool)
            n668 = case shown="True" w973 {
              frame False {
              }
              frame True {
                n669 = stacked-sequence {
                  seq-local: [w974 _ _] -> [_ w976 _]
                  frame #0 {
                    n670 = call "CALIBRATION PASSWORD"() -> ("PASSWORD"=w974:string)  [unwired: 17 in, 2 out]
                  }
                  frame #1 {
                    n671 = Equal?(x=w976, y="7777") -> (x = y?=w975:bool)
                    n672 = case shown="True" w975 {
                      frame False {
                      }
                      frame True {
                        n673 = stacked-sequence {
                          frame #0 {
                            n674 = call "sub vi - calibration v1.vi"() -> ()  [unwired: 12 in]
                          }
                          frame #1 {
                            n675 = call "sub vi - get calibration values v1.vi"() -> ("LAB01 (CAL)"=w982:T7, "LAB02 (CAL)"=w981:T8, "LAB03 (CAL)"=w980:T7, "LAB04 (CAL)"=w979:T7, "calibration file error out"=w983:errorcluster, "LAB05 (CAL)"=w978:T7)  [unwired: 10 in]
                            n676 = local write "calibration file error out"(w983) -> ()
                            n677 = local write "LAB04 (CAL)"(w979) -> ()
                            n678 = local write "LAB05 (CAL)"(w978) -> ()
                            n679 = local write "LAB01 (CAL)"(w982) -> ()
                            n680 = local write "LAB02 (CAL)"(w981) -> ()
                            n681 = local write "LAB03 (CAL)"(w980) -> ()
                          }
                        }
                      }
                    }
                  }
                  frame #2 {
                    n682 = local write "CALIBRATE"(FALSE) -> ()
                  }
                }
              }
            }
          }
        }
        n683 = node-c288() -> ()  [unwired: 1 in, 1 out]
        "loops" <- w24
      }
      n684 = node-c288(w10) -> ()  [unwired: 1 out]
    }
  }
